vi "[File Management] - PC Module.vi"() -> ()   [LabVIEW 2020]
uses:
  Utility/TypeDefs_Utility/ENUM RB_Pos_Quadrant Position.ctl
  TypeDefs/ENUM_Request PC File Manager.ctl
  TypeDefs/ENUM_State PC File Manager.ctl
  Utility/FP/FPClass/DecFrame_FP/DecFrame_FP.lvclass
  <vilib>/Utility/error.llb/DialogType.ctl
  facef2d7-9603-4ff4-9ff0-56512382c7b7.vi
  d08d4191-17b2-482f-a441-d9d60e68be63.vi
  a00c5825-d05e-4c72-92a9-d0f4f7d392b7.vi
  f268d36e-7cae-4eee-81c7-8a8159c411db.vi
  ade89b95-2dfa-48cf-afe4-b6056d13f73a.vi
  2597e34f-0f19-4283-a693-10768823b2c8.vi
  06699f3f-2e82-4b79-aa69-334e1d5944f8.vi
  <vilib>/Rock Robotics/WPI/ThirdParty/Phoenix-LabVIEW/Motor Controller/Controls/CTRE_Phoenix_MotorControl_TalonFXInvertType.ctl
  Shared Code/TypeDefs/Cluster_Enable-Value DBL.ctl
  <vilib>/Rock Robotics/WPI/ThirdParty/Phoenix-LabVIEW/Motor Controller/Controls/CTRE_Phoenix_MotorControl_NeutralMode.ctl
  Shared Code/TypeDefs/Cluster_Swerve Module Drive Config Data.ctl
  Shared Code/TypeDefs/Cluster_Motion Magic Parameters.ctl
  Shared Code/TypeDefs/Cluster_Swerve Module Azimuth Config Data.ctl
  316f2880-b704-4a84-a7ff-cf39f3abe56d.vi
  f9576979-38bd-4a02-92ac-858de525dc8c.vi
  <vilib>/WebDAVClient/NI_WebDAV.lvlib
  <vilib>/WebDAVClient/Advanced/SessionHandle.ctl
  Shared Code/TypeDefs/Cluster_High-Low.ctl
  Shared Code/TypeDefs/Cluster_PID Gains.ctl
  Shared Code/TypeDefs/Cluster_PID Config.ctl
  Shared Code/TypeDefs/Cluster_Sholder_Config HW Values.ctl
  Shared Code/TypeDefs/Cluster_Extend_Config HW Values.ctl
  Shared Code/TypeDefs/Cluster_Wrist_Config HW Values.ctl
  Shared Code/TypeDefs/ENUM_Motor Index.ctl
  Shared Code/TypeDefs/Cluster_Module Specific Config Data.ctl
  Shared Code/TypeDefs/Cluster_Swerve Specific Data.ctl
  8aa61b50-d4c1-4d7c-b518-7e7f89ee47b3.vi
  293a5106-20bb-4168-be9a-18547983b4f2.vi
  ae0c41dc-fba3-4b78-a09b-fb6d66dd20f7.vi
  fc6d8c50-d7f1-4b91-8983-8391aab75057.vi
  d093f6e5-c98f-44c5-8e41-37ffdc5fbdf3.vi
  Shared Code/TypeDefs/Cluster_Grabber_Config FX Values.ctl
  3a4f407e-2c67-43cb-a4fb-f8418298715f.vi
  <vilib>/WebDAVClient/Advanced/FileInfo.ctl
  d1a17949-e99a-4e11-84fa-4c63115c30d4.vi
  7235e565-7edd-4e1e-80f2-698df6b339dd.vi
  135ee32a-b968-4bc4-aa5f-92b1bd27fa7a.vi
  d92062e0-e931-44ed-a5ae-2fad103b160f.vi
  392f1fec-bdba-4268-92de-5fc60040c1a5.vi
  5390630c-9484-4680-9f8f-9f3095daa9a3.vi
  8e06bce4-31bf-4e2c-9356-0233bb58fc1e.vi
  8021acdc-735e-4c3a-8370-c2cd77d975ff.vi
  fe44edcd-002d-483e-8bc4-2119d9f98af6.vi
  213a5e39-b7ba-45fa-89ff-ac0bf8954cfe.vi
  32e82365-4a9b-4a03-b1c6-655977ec55ce.vi
  6dfe48be-dd7d-41aa-9213-7bde1fbabe93.vi
  ec83e26c-9f45-47fe-bb3a-23606bf88b00.vi
  fc97c97f-c470-4d18-867d-310d18e3dab9.vi
  6ebbc37a-f38e-4f02-af33-7071d1f24c56.vi
  bb6ae5b7-7e89-4e26-bd0e-9cffb8a8ccf7.vi
  Shared Code/TypeDefs/Cluster_FWD  REV Values.ctl
  Shared Code/TypeDefs/Cluster_Config Motor Output.ctl
  Shared Code/TypeDefs/Cluser_Enable-Value I32.ctl
  Shared Code/TypeDefs/Cluser_Config_Soft Limits.ctl
  <vilib>/Rock Robotics/WPI/ThirdParty/Phoenix-LabVIEW/Motor Controller/Controls/CTRE_Phoenix_MotorControl_LimitSwitchNormal.ctl
  Shared Code/TypeDefs/Cluser_Hard Limits.ctl
  Shared Code/TypeDefs/Cluser_Limit Travel Config.ctl
  Shared Code/TypeDefs/Cluser_CAN Data.ctl
  Shared Code/TypeDefs/Cluster_Extend_Config SW Values.ctl
  Shared Code/TypeDefs/Cluser_Config_Current Limits.ctl
  Shared Code/TypeDefs/Cluster_Config_Cancoder Data.ctl
  33df8094-f942-4665-8c4a-d95e8868fd54.vi
  1feea5ea-1d58-47d3-a6aa-f7318612a923.vi
  Shared Code/TypeDefs/ENUM_AutoSelect.ctl
  roboRIO Code/Systems/AUTO 2023/ENUM_CMD_State.ctl
  roboRIO Code/Systems/AUTO 2023/2023-Auto_CMD.lvlib
  roboRIO Code/Systems/AUTO 2023/ENUM_Drive Mode Select.ctl
  Shared Code/TypeDefs/ENUM_Grabber_CMD_Mode Select.ctl
  roboRIO Code/Systems/MotionMaser/ENUM_Pose List.ctl
  roboRIO Code/Systems/MotionMaser/MotionMaster_SubCMD.lvlib
  Shared Code/TypeDefs/Dial_Compase heading unit circle CCW positive.ctl
  Shared Code/TypeDefs/Cluster_Auto Sequence Settings.ctl
  Shared Code/TypeDefs/Cluster_Auto Sequence Data.ctl
  Shared Code/TypeDefs/Cluster_AutoSequence.ctl
  Shared Code/TypeDefs/Cluster_Config_AutoData.ctl
panel:
  in  "AutoData":T1 {"Sequences"."List"."CMDs"."Auto Angle" scale format="%.3f"}
  out "Config NOT Equal":bool
  out "PC Config NOT Saved":bool
  in  "Save RIO Config":bool
  in  "Save PC Config":bool
  in  "Read RIO Config":bool
  in  "Read PC Config":bool
  in  "Copy RIO to PC":bool
  in  "Copy PC to RIO":bool
  in  "Config Tab":T11(tab)
  in  "PC Module Specific Data":T12={"SpecificData Ver"=0, "Data"=[{"Motor Pos"=enum."Left-Front", "CAN Bus"="", "Drive ID"=5, "Azimuth ID"=1, "CanCoder ID"=1, "CanCoder Offset"=14.502}, {"Motor Pos"=enum."Right-Front", "CAN Bus"="", "Drive ID"=6, "Azimuth ID"=2, "CanCoder ID"=2, "CanCoder Offset"=166.816}, {"Motor Pos"=enum."Right-Back", "CAN Bus"="", "Drive ID"=7, "Azimuth ID"=3, "CanCoder ID"=3, "CanCoder Offset"=50.273}, {"Motor Pos"=enum."Left-Back", "CAN Bus"="", "Drive ID"=8, "Azimuth ID"=4, "CanCoder ID"=4, "CanCoder Offset"=332.842}]}
  out "RIO Module Specific Data":T12={"SpecificData Ver"=0, "Data"=[{"Motor Pos"=enum."Left-Front", "CAN Bus"="", "Drive ID"=5, "Azimuth ID"=1, "CanCoder ID"=1, "CanCoder Offset"=14.502}, {"Motor Pos"=enum."Right-Front", "CAN Bus"="", "Drive ID"=6, "Azimuth ID"=2, "CanCoder ID"=2, "CanCoder Offset"=166.816}, {"Motor Pos"=enum."Right-Back", "CAN Bus"="", "Drive ID"=7, "Azimuth ID"=3, "CanCoder ID"=3, "CanCoder Offset"=50.273}, {"Motor Pos"=enum."Left-Back", "CAN Bus"="", "Drive ID"=8, "Azimuth ID"=4, "CanCoder ID"=4, "CanCoder Offset"=332.842}]}
  in  "PC Azimuth Config Data":T15={"ModuleAzimuth Ver"=0, "Output"={"Type"=enum."Clockwise", "Neutral"=enum."Override to Brake", "Max"={"FWD"=0.0, "REV"=2.0}, "Min"={"FWD"=0.0, "REV"=0.0}, "OL Ramp Rate (S)"=0.0, "Dead Band"=0.0}, "CL"={"Gains"={"P"=0.0, "I"=0.0, "D"=20.0, "F"=0.0}, "Error Allowed"={"High"=0.0, "Low"=0.0}, "I Zone"={"High"=0.0, "Low"=0.0}, "Max Out"={"FWD"=20.0, "REV"=0.0}, "Max I Accu"={"High"=1.0, "Low"=-1.0}, "CL Ramp Rate (S)"=0.0}, "MM"={"Cruise Velocity"=0, "Acceleration"=0}} {"Output"."Min"."REV" format="%.2f"; "Output"."Min"."FWD" format="%.2f"; "Output"."Max"."REV" format="%.2f"; "Output"."Max"."FWD" format="%.2f"; "CL"."Max I Accu"."Low" format="%#.8f"; "CL"."Max I Accu"."High" format="%#.8f"; "CL"."Gains"."F" format="%#.8f"; "CL"."Gains"."D" format="%#.8f"; "CL"."Gains"."I" format="%#.8f"; "CL"."Gains"."P" format="%#.8f"; "CL"."Error Allowed"."Low" format="%#.8f"; "CL"."Error Allowed"."High" format="%#.8f"; "CL"."I Zone"."Low" format="%#.8f"; "CL"."I Zone"."High" format="%#.8f"; "CL"."Max Out"."REV" format="%.2f"; "CL"."Max Out"."FWD" format="%.2f"}
  out "RIO Azimuth Config Data":T15={"ModuleAzimuth Ver"=0, "Output"={"Type"=enum."Clockwise", "Neutral"=enum."Override to Brake", "Max"={"FWD"=0.0, "REV"=2.0}, "Min"={"FWD"=0.0, "REV"=0.0}, "OL Ramp Rate (S)"=0.0, "Dead Band"=0.0}, "CL"={"Gains"={"P"=0.0, "I"=0.0, "D"=20.0, "F"=0.0}, "Error Allowed"={"High"=0.0, "Low"=0.0}, "I Zone"={"High"=0.0, "Low"=0.0}, "Max Out"={"FWD"=20.0, "REV"=0.0}, "Max I Accu"={"High"=1.0, "Low"=-1.0}, "CL Ramp Rate (S)"=0.0}, "MM"={"Cruise Velocity"=0, "Acceleration"=0}} {"Output"."Min"."REV" format="%.2f"; "Output"."Min"."FWD" format="%.2f"; "Output"."Max"."REV" format="%.2f"; "Output"."Max"."FWD" format="%.2f"; "CL"."Max I Accu"."Low" format="%#.8f"; "CL"."Max I Accu"."High" format="%#.8f"; "CL"."Gains"."F" format="%#.8f"; "CL"."Gains"."D" format="%#.8f"; "CL"."Gains"."I" format="%#.8f"; "CL"."Gains"."P" format="%#.8f"; "CL"."Error Allowed"."Low" format="%#.8f"; "CL"."Error Allowed"."High" format="%#.8f"; "CL"."I Zone"."Low" format="%#.8f"; "CL"."I Zone"."High" format="%#.8f"; "CL"."Max Out"."REV" format="%.2f"; "CL"."Max Out"."FWD" format="%.2f"}
  in  "PC Drive Config Data":T24={"ModuleDrive Ver"=0, "Output"={"Type"=enum."Counter-Clockwise", "Neutral"=enum."EEPROMSetting", "Max"={"FWD"=0.0, "REV"=0.0}, "Min"={"FWD"=0.0, "REV"=0.0}, "OL Ramp Rate (S)"=0.0, "Dead Band"=0.0}, "CL"={"Gains"={"P"=1.0, "I"=0.01, "D"=0.0, "F"=0.0}, "Error Allowed"={"High"=0.1, "Low"=-0.1}, "I Zone"={"High"=10.0, "Low"=-10.0}, "Max Out"={"FWD"=100.0, "REV"=-100.0}, "Max I Accu"={"High"=0.0, "Low"=0.0}, "CL Ramp Rate (S)"=0.0}, "VoltageComp"={"Enable"=FALSE, "Value"=0.0}} {"Output"."Min"."REV" format="%.2f"; "Output"."Min"."FWD" format="%.2f"; "Output"."Max"."REV" format="%.2f"; "Output"."Max"."FWD" format="%.2f"; "VoltageComp"."Value" format="%.1g"; "CL"."Max I Accu"."Low" format="%#.8f"; "CL"."Max I Accu"."High" format="%#.8f"; "CL"."Gains"."F" format="%#.8f"; "CL"."Gains"."D" format="%#.8f"; "CL"."Gains"."I" format="%#.8f"; "CL"."Gains"."P" format="%#.8f"; "CL"."Error Allowed"."Low" format="%#.8f"; "CL"."Error Allowed"."High" format="%#.8f"; "CL"."I Zone"."Low" format="%#.8f"; "CL"."I Zone"."High" format="%#.8f"; "CL"."Max Out"."REV" format="%.2f"; "CL"."Max Out"."FWD" format="%.2f"}
  out "RIO Drive Config Data":T24={"ModuleDrive Ver"=0, "Output"={"Type"=enum."Counter-Clockwise", "Neutral"=enum."EEPROMSetting", "Max"={"FWD"=0.0, "REV"=0.0}, "Min"={"FWD"=0.0, "REV"=0.0}, "OL Ramp Rate (S)"=0.0, "Dead Band"=0.0}, "CL"={"Gains"={"P"=1.0, "I"=0.01, "D"=0.0, "F"=0.0}, "Error Allowed"={"High"=0.1, "Low"=-0.1}, "I Zone"={"High"=10.0, "Low"=-10.0}, "Max Out"={"FWD"=100.0, "REV"=-100.0}, "Max I Accu"={"High"=0.0, "Low"=0.0}, "CL Ramp Rate (S)"=0.0}, "VoltageComp"={"Enable"=FALSE, "Value"=0.0}} {"Output"."Min"."REV" format="%.2f"; "Output"."Min"."FWD" format="%.2f"; "Output"."Max"."REV" format="%.2f"; "Output"."Max"."FWD" format="%.2f"; "VoltageComp"."Value" format="%.1g"; "CL"."Max I Accu"."Low" format="%#.8f"; "CL"."Max I Accu"."High" format="%#.8f"; "CL"."Gains"."F" format="%#.8f"; "CL"."Gains"."D" format="%#.8f"; "CL"."Gains"."I" format="%#.8f"; "CL"."Gains"."P" format="%#.8f"; "CL"."Error Allowed"."Low" format="%#.8f"; "CL"."Error Allowed"."High" format="%#.8f"; "CL"."I Zone"."Low" format="%#.8f"; "CL"."I Zone"."High" format="%#.8f"; "CL"."Max Out"."REV" format="%.2f"; "CL"."Max Out"."FWD" format="%.2f"}
  in  "PC Sholder Config":T26={"SholderHW Ver"=0, "CAN"={"ID"=0, "Bus"=""}, "Output"={"Type"=enum."Counter-Clockwise", "Neutral"=enum."Override to Brake", "Max"={"FWD"=0.0, "REV"=-1.0}, "Min"={"FWD"=0.0, "REV"=0.0}, "OL Ramp Rate (S)"=0.0, "Dead Band"=0.0}, "CL"={"Gains"={"P"=1.0, "I"=0.01, "D"=0.0, "F"=0.0}, "Error Allowed"={"High"=0.0, "Low"=0.0}, "I Zone"={"High"=10000.0, "Low"=-1000.0}, "Max Out"={"FWD"=1.0, "REV"=-1.0}, "Max I Accu"={"High"=10.0, "Low"=-10.0}, "CL Ramp Rate (S)"=0.0}, "MM"={"Cruise Velocity"=5000, "Acceleration"=5000}, "TravelLimits"={"Hard"={"FWD Switch Normal"=enum."Normally Open", "FWD On will Zero Encoder "=FALSE, "REV Switch Normal"=enum."Normally Open", "REV On will Zero Encoder "=FALSE}, "Soft"={"FWD"={"Enable"=FALSE, "Counts"=0}, "REV"={"Enable"=FALSE, "Counts"=0}}}, "Cancoder"={"ID"=0, "CW(t) CCW(f)"=TRUE, "Zero Offset"=0.0}} {"TravelLimits"."Soft"."REV"."Counts" format="%#.0f"; "TravelLimits"."Soft"."FWD"."Counts" format="%#.0f"; "Output"."Min"."REV" format="%.2f"; "Output"."Min"."FWD" format="%.2f"; "Output"."Max"."REV" format="%.2f"; "Output"."Max"."FWD" format="%.2f"; "CL"."Max I Accu"."Low" format="%#.8f"; "CL"."Max I Accu"."High" format="%#.8f"; "CL"."Gains"."F" format="%#.8f"; "CL"."Gains"."D" format="%#.8f"; "CL"."Gains"."I" format="%#.8f"; "CL"."Gains"."P" format="%#.8f"; "CL"."Error Allowed"."Low" format="%#.8f"; "CL"."Error Allowed"."High" format="%#.8f"; "CL"."I Zone"."Low" format="%#.8f"; "CL"."I Zone"."High" format="%#.8f"; "CL"."Max Out"."REV" format="%.2f"; "CL"."Max Out"."FWD" format="%.2f"}
  out "RIO Sholder Config":T26={"SholderHW Ver"=0, "CAN"={"ID"=0, "Bus"=""}, "Output"={"Type"=enum."Counter-Clockwise", "Neutral"=enum."Override to Brake", "Max"={"FWD"=0.0, "REV"=-1.0}, "Min"={"FWD"=0.0, "REV"=0.0}, "OL Ramp Rate (S)"=0.0, "Dead Band"=0.0}, "CL"={"Gains"={"P"=1.0, "I"=0.01, "D"=0.0, "F"=0.0}, "Error Allowed"={"High"=0.0, "Low"=0.0}, "I Zone"={"High"=10000.0, "Low"=-1000.0}, "Max Out"={"FWD"=1.0, "REV"=-1.0}, "Max I Accu"={"High"=10.0, "Low"=-10.0}, "CL Ramp Rate (S)"=0.0}, "MM"={"Cruise Velocity"=5000, "Acceleration"=5000}, "TravelLimits"={"Hard"={"FWD Switch Normal"=enum."Normally Open", "FWD On will Zero Encoder "=FALSE, "REV Switch Normal"=enum."Normally Open", "REV On will Zero Encoder "=FALSE}, "Soft"={"FWD"={"Enable"=FALSE, "Counts"=0}, "REV"={"Enable"=FALSE, "Counts"=0}}}, "Cancoder"={"ID"=0, "CW(t) CCW(f)"=TRUE, "Zero Offset"=0.0}} {"TravelLimits"."Soft"."REV"."Counts" format="%#.0f"; "TravelLimits"."Soft"."FWD"."Counts" format="%#.0f"; "Output"."Min"."REV" format="%.2f"; "Output"."Min"."FWD" format="%.2f"; "Output"."Max"."REV" format="%.2f"; "Output"."Max"."FWD" format="%.2f"; "CL"."Max I Accu"."Low" format="%#.8f"; "CL"."Max I Accu"."High" format="%#.8f"; "CL"."Gains"."F" format="%#.8f"; "CL"."Gains"."D" format="%#.8f"; "CL"."Gains"."I" format="%#.8f"; "CL"."Gains"."P" format="%#.8f"; "CL"."Error Allowed"."Low" format="%#.8f"; "CL"."Error Allowed"."High" format="%#.8f"; "CL"."I Zone"."Low" format="%#.8f"; "CL"."I Zone"."High" format="%#.8f"; "CL"."Max Out"."REV" format="%.2f"; "CL"."Max Out"."FWD" format="%.2f"}
  in  "PC Extend ConfigFX":T34={"ExtendHW Ver"=0, "CAN"={"ID"=0, "Bus"=""}, "Output"={"Type"=enum."Counter-Clockwise", "Neutral"=enum."Override to Brake", "Max"={"FWD"=0.0, "REV"=-1.0}, "Min"={"FWD"=0.0, "REV"=0.0}, "OL Ramp Rate (S)"=0.0, "Dead Band"=0.0}, "CL"={"Gains"={"P"=1.0, "I"=0.01, "D"=0.0, "F"=0.0}, "Error Allowed"={"High"=0.0, "Low"=0.0}, "I Zone"={"High"=10000.0, "Low"=-1000.0}, "Max Out"={"FWD"=1.0, "REV"=-1.0}, "Max I Accu"={"High"=10.0, "Low"=-10.0}, "CL Ramp Rate (S)"=0.0}, "MM"={"Cruise Velocity"=5000, "Acceleration"=5000}, "TravelLimits"={"Hard"={"FWD Switch Normal"=enum."Normally Open", "FWD On will Zero Encoder "=FALSE, "REV Switch Normal"=enum."Normally Open", "REV On will Zero Encoder "=FALSE}, "Soft"={"FWD"={"Enable"=FALSE, "Counts"=0}, "REV"={"Enable"=FALSE, "Counts"=0}}}, "StatorLimit"={"Enable"=FALSE, "Current Limit"=0.0, "Threshold Current"=0.0, "Threshold Time"=0.0}, "Cancoder"={"ID"=0, "CW(t) CCW(f)"=FALSE, "Zero Offset"=0.0}} {"TravelLimits"."Soft"."REV"."Counts" format="%#.0f"; "TravelLimits"."Soft"."FWD"."Counts" format="%#.0f"; "Output"."Min"."REV" format="%.2f"; "Output"."Min"."FWD" format="%.2f"; "Output"."Max"."REV" format="%.2f"; "Output"."Max"."FWD" format="%.2f"; "CL"."Max I Accu"."Low" format="%#.8f"; "CL"."Max I Accu"."High" format="%#.8f"; "CL"."Gains"."F" format="%#.8f"; "CL"."Gains"."D" format="%#.8f"; "CL"."Gains"."I" format="%#.8f"; "CL"."Gains"."P" format="%#.8f"; "CL"."Error Allowed"."Low" format="%#.8f"; "CL"."Error Allowed"."High" format="%#.8f"; "CL"."I Zone"."Low" format="%#.8f"; "CL"."I Zone"."High" format="%#.8f"; "CL"."Max Out"."REV" format="%.2f"; "CL"."Max Out"."FWD" format="%.2f"}
  out "RIO Extender Config":T34={"ExtendHW Ver"=0, "CAN"={"ID"=0, "Bus"=""}, "Output"={"Type"=enum."Counter-Clockwise", "Neutral"=enum."Override to Brake", "Max"={"FWD"=0.0, "REV"=-1.0}, "Min"={"FWD"=0.0, "REV"=0.0}, "OL Ramp Rate (S)"=0.0, "Dead Band"=0.0}, "CL"={"Gains"={"P"=1.0, "I"=0.01, "D"=0.0, "F"=0.0}, "Error Allowed"={"High"=0.0, "Low"=0.0}, "I Zone"={"High"=10000.0, "Low"=-1000.0}, "Max Out"={"FWD"=1.0, "REV"=-1.0}, "Max I Accu"={"High"=10.0, "Low"=-10.0}, "CL Ramp Rate (S)"=0.0}, "MM"={"Cruise Velocity"=5000, "Acceleration"=5000}, "TravelLimits"={"Hard"={"FWD Switch Normal"=enum."Normally Open", "FWD On will Zero Encoder "=FALSE, "REV Switch Normal"=enum."Normally Open", "REV On will Zero Encoder "=FALSE}, "Soft"={"FWD"={"Enable"=FALSE, "Counts"=0}, "REV"={"Enable"=FALSE, "Counts"=0}}}, "StatorLimit"={"Enable"=FALSE, "Current Limit"=0.0, "Threshold Current"=0.0, "Threshold Time"=0.0}, "Cancoder"={"ID"=0, "CW(t) CCW(f)"=FALSE, "Zero Offset"=0.0}} {"TravelLimits"."Soft"."REV"."Counts" format="%#.0f"; "TravelLimits"."Soft"."FWD"."Counts" format="%#.0f"; "Output"."Min"."REV" format="%.2f"; "Output"."Min"."FWD" format="%.2f"; "Output"."Max"."REV" format="%.2f"; "Output"."Max"."FWD" format="%.2f"; "CL"."Max I Accu"."Low" format="%#.8f"; "CL"."Max I Accu"."High" format="%#.8f"; "CL"."Gains"."F" format="%#.8f"; "CL"."Gains"."D" format="%#.8f"; "CL"."Gains"."I" format="%#.8f"; "CL"."Gains"."P" format="%#.8f"; "CL"."Error Allowed"."Low" format="%#.8f"; "CL"."Error Allowed"."High" format="%#.8f"; "CL"."I Zone"."Low" format="%#.8f"; "CL"."I Zone"."High" format="%#.8f"; "CL"."Max Out"."REV" format="%.2f"; "CL"."Max Out"."FWD" format="%.2f"}
  in  "PC Wrist Config":T36={"WristHW Ver"=0, "CAN"={"ID"=0, "Bus"=""}, "Output"={"Type"=enum."Counter-Clockwise", "Neutral"=enum."Override to Brake", "Max"={"FWD"=0.0, "REV"=-1.0}, "Min"={"FWD"=0.0, "REV"=0.0}, "OL Ramp Rate (S)"=0.0, "Dead Band"=0.0}, "CL"={"Gains"={"P"=1.0, "I"=0.01, "D"=0.0, "F"=0.0}, "Error Allowed"={"High"=0.0, "Low"=0.0}, "I Zone"={"High"=10000.0, "Low"=-1000.0}, "Max Out"={"FWD"=1.0, "REV"=-1.0}, "Max I Accu"={"High"=10.0, "Low"=-10.0}, "CL Ramp Rate (S)"=0.0}, "MM"={"Cruise Velocity"=5000, "Acceleration"=5000}, "TravelLimits"={"Hard"={"FWD Switch Normal"=enum."Normally Open", "FWD On will Zero Encoder "=FALSE, "REV Switch Normal"=enum."Normally Open", "REV On will Zero Encoder "=FALSE}, "Soft"={"FWD"={"Enable"=FALSE, "Counts"=0}, "REV"={"Enable"=FALSE, "Counts"=0}}}, "Cancoder"={"ID"=0, "CW(t) CCW(f)"=TRUE, "Zero Offset"=0.0}, "CurrentLimit"={"Enable"=FALSE, "Current Limit"=0.0, "Threshold Current"=0.0, "Threshold Time"=0.0}} {"TravelLimits"."Soft"."REV"."Counts" format="%#.0f"; "TravelLimits"."Soft"."FWD"."Counts" format="%#.0f"; "Output"."Min"."REV" format="%.2f"; "Output"."Min"."FWD" format="%.2f"; "Output"."Max"."REV" format="%.2f"; "Output"."Max"."FWD" format="%.2f"; "CL"."Max I Accu"."Low" format="%#.8f"; "CL"."Max I Accu"."High" format="%#.8f"; "CL"."Gains"."F" format="%#.8f"; "CL"."Gains"."D" format="%#.8f"; "CL"."Gains"."I" format="%#.8f"; "CL"."Gains"."P" format="%#.8f"; "CL"."Error Allowed"."Low" format="%#.8f"; "CL"."Error Allowed"."High" format="%#.8f"; "CL"."I Zone"."Low" format="%#.8f"; "CL"."I Zone"."High" format="%#.8f"; "CL"."Max Out"."REV" format="%.2f"; "CL"."Max Out"."FWD" format="%.2f"}
  out "RIO Wrist Config":T36={"WristHW Ver"=0, "CAN"={"ID"=0, "Bus"=""}, "Output"={"Type"=enum."Counter-Clockwise", "Neutral"=enum."Override to Brake", "Max"={"FWD"=0.0, "REV"=-1.0}, "Min"={"FWD"=0.0, "REV"=0.0}, "OL Ramp Rate (S)"=0.0, "Dead Band"=0.0}, "CL"={"Gains"={"P"=1.0, "I"=0.01, "D"=0.0, "F"=0.0}, "Error Allowed"={"High"=0.0, "Low"=0.0}, "I Zone"={"High"=10000.0, "Low"=-1000.0}, "Max Out"={"FWD"=1.0, "REV"=-1.0}, "Max I Accu"={"High"=10.0, "Low"=-10.0}, "CL Ramp Rate (S)"=0.0}, "MM"={"Cruise Velocity"=5000, "Acceleration"=5000}, "TravelLimits"={"Hard"={"FWD Switch Normal"=enum."Normally Open", "FWD On will Zero Encoder "=FALSE, "REV Switch Normal"=enum."Normally Open", "REV On will Zero Encoder "=FALSE}, "Soft"={"FWD"={"Enable"=FALSE, "Counts"=0}, "REV"={"Enable"=FALSE, "Counts"=0}}}, "Cancoder"={"ID"=0, "CW(t) CCW(f)"=TRUE, "Zero Offset"=0.0}, "CurrentLimit"={"Enable"=FALSE, "Current Limit"=0.0, "Threshold Current"=0.0, "Threshold Time"=0.0}} {"TravelLimits"."Soft"."REV"."Counts" format="%#.0f"; "TravelLimits"."Soft"."FWD"."Counts" format="%#.0f"; "Output"."Min"."REV" format="%.2f"; "Output"."Min"."FWD" format="%.2f"; "Output"."Max"."REV" format="%.2f"; "Output"."Max"."FWD" format="%.2f"; "CL"."Max I Accu"."Low" format="%#.8f"; "CL"."Max I Accu"."High" format="%#.8f"; "CL"."Gains"."F" format="%#.8f"; "CL"."Gains"."D" format="%#.8f"; "CL"."Gains"."I" format="%#.8f"; "CL"."Gains"."P" format="%#.8f"; "CL"."Error Allowed"."Low" format="%#.8f"; "CL"."Error Allowed"."High" format="%#.8f"; "CL"."I Zone"."Low" format="%#.8f"; "CL"."I Zone"."High" format="%#.8f"; "CL"."Max Out"."REV" format="%.2f"; "CL"."Max Out"."FWD" format="%.2f"}
  in  "PC ExtendProgram Config":T37={"ExtendSW Ver"=0, "Home Speed (0-1)"=0.0, "Enable Current Limit On Homing"=FALSE, "At Position Delay(S)"=0.2}
  out "RIO ExtendProgram Config":T37={"ExtendSW Ver"=0, "Home Speed (0-1)"=0.0, "Enable Current Limit On Homing"=FALSE, "At Position Delay(S)"=0.2}
  in  "PC Grabber Config":T38={"Grabber Ver"=0, "CAN"={"ID"=136, "Bus"=""}, "Output"={"Type"=enum."Counter-Clockwise", "Neutral"=enum."Override to Brake", "Max"={"FWD"=0.0, "REV"=5000.0}, "Min"={"FWD"=0.0, "REV"=0.0}, "OL Ramp Rate (S)"=0.0, "Dead Band"=0.0}, "StatorLimit"={"Enable"=FALSE, "Current Limit"=0.0, "Threshold Current"=0.0, "Threshold Time"=0.0}} {"Output"."Min"."REV" format="%.2f"; "Output"."Min"."FWD" format="%.2f"; "Output"."Max"."REV" format="%.2f"; "Output"."Max"."FWD" format="%.2f"}
  out "RIO Grabber Config":T38={"Grabber Ver"=0, "CAN"={"ID"=136, "Bus"=""}, "Output"={"Type"=enum."Counter-Clockwise", "Neutral"=enum."Override to Brake", "Max"={"FWD"=0.0, "REV"=5000.0}, "Min"={"FWD"=0.0, "REV"=0.0}, "OL Ramp Rate (S)"=0.0, "Dead Band"=0.0}, "StatorLimit"={"Enable"=FALSE, "Current Limit"=0.0, "Threshold Current"=0.0, "Threshold Time"=0.0}} {"Output"."Min"."REV" format="%.2f"; "Output"."Min"."FWD" format="%.2f"; "Output"."Max"."REV" format="%.2f"; "Output"."Max"."FWD" format="%.2f"}
  out "PC Folder Found":bool
  out "RIO Folder Found":bool
  out "RIO Connected":bool
  out "PC Folder Path":path
  in  "RIO Folder Path":string
  in  "Select":bool[](array[boolean])
  in  "RIO IP List":string[](array[string])
  out "Message":string
  in  "stop":bool
  out "Action":string
  out "Next Request":T39 caption="Request"
  out "State":T40=enum."Connecting to RIO"
  # "Tune Output\nto 1023 Max"
  # "Tune Output\nto 1023 Max"
  # "Tune to Output\nto 1023 Max"
  # "Tune to Output\nto 1023 Max"
  # "Tune Output\nto 1023 Max"
  # "Tune Output\nto 1023 Max"
  # "Tune Output\nto 1023 Max"
  # "Tune Output\nto 1023 Max"
  # "Tune Output\nto 1023 Max"
  # "Tune Output\nto 1023 Max"
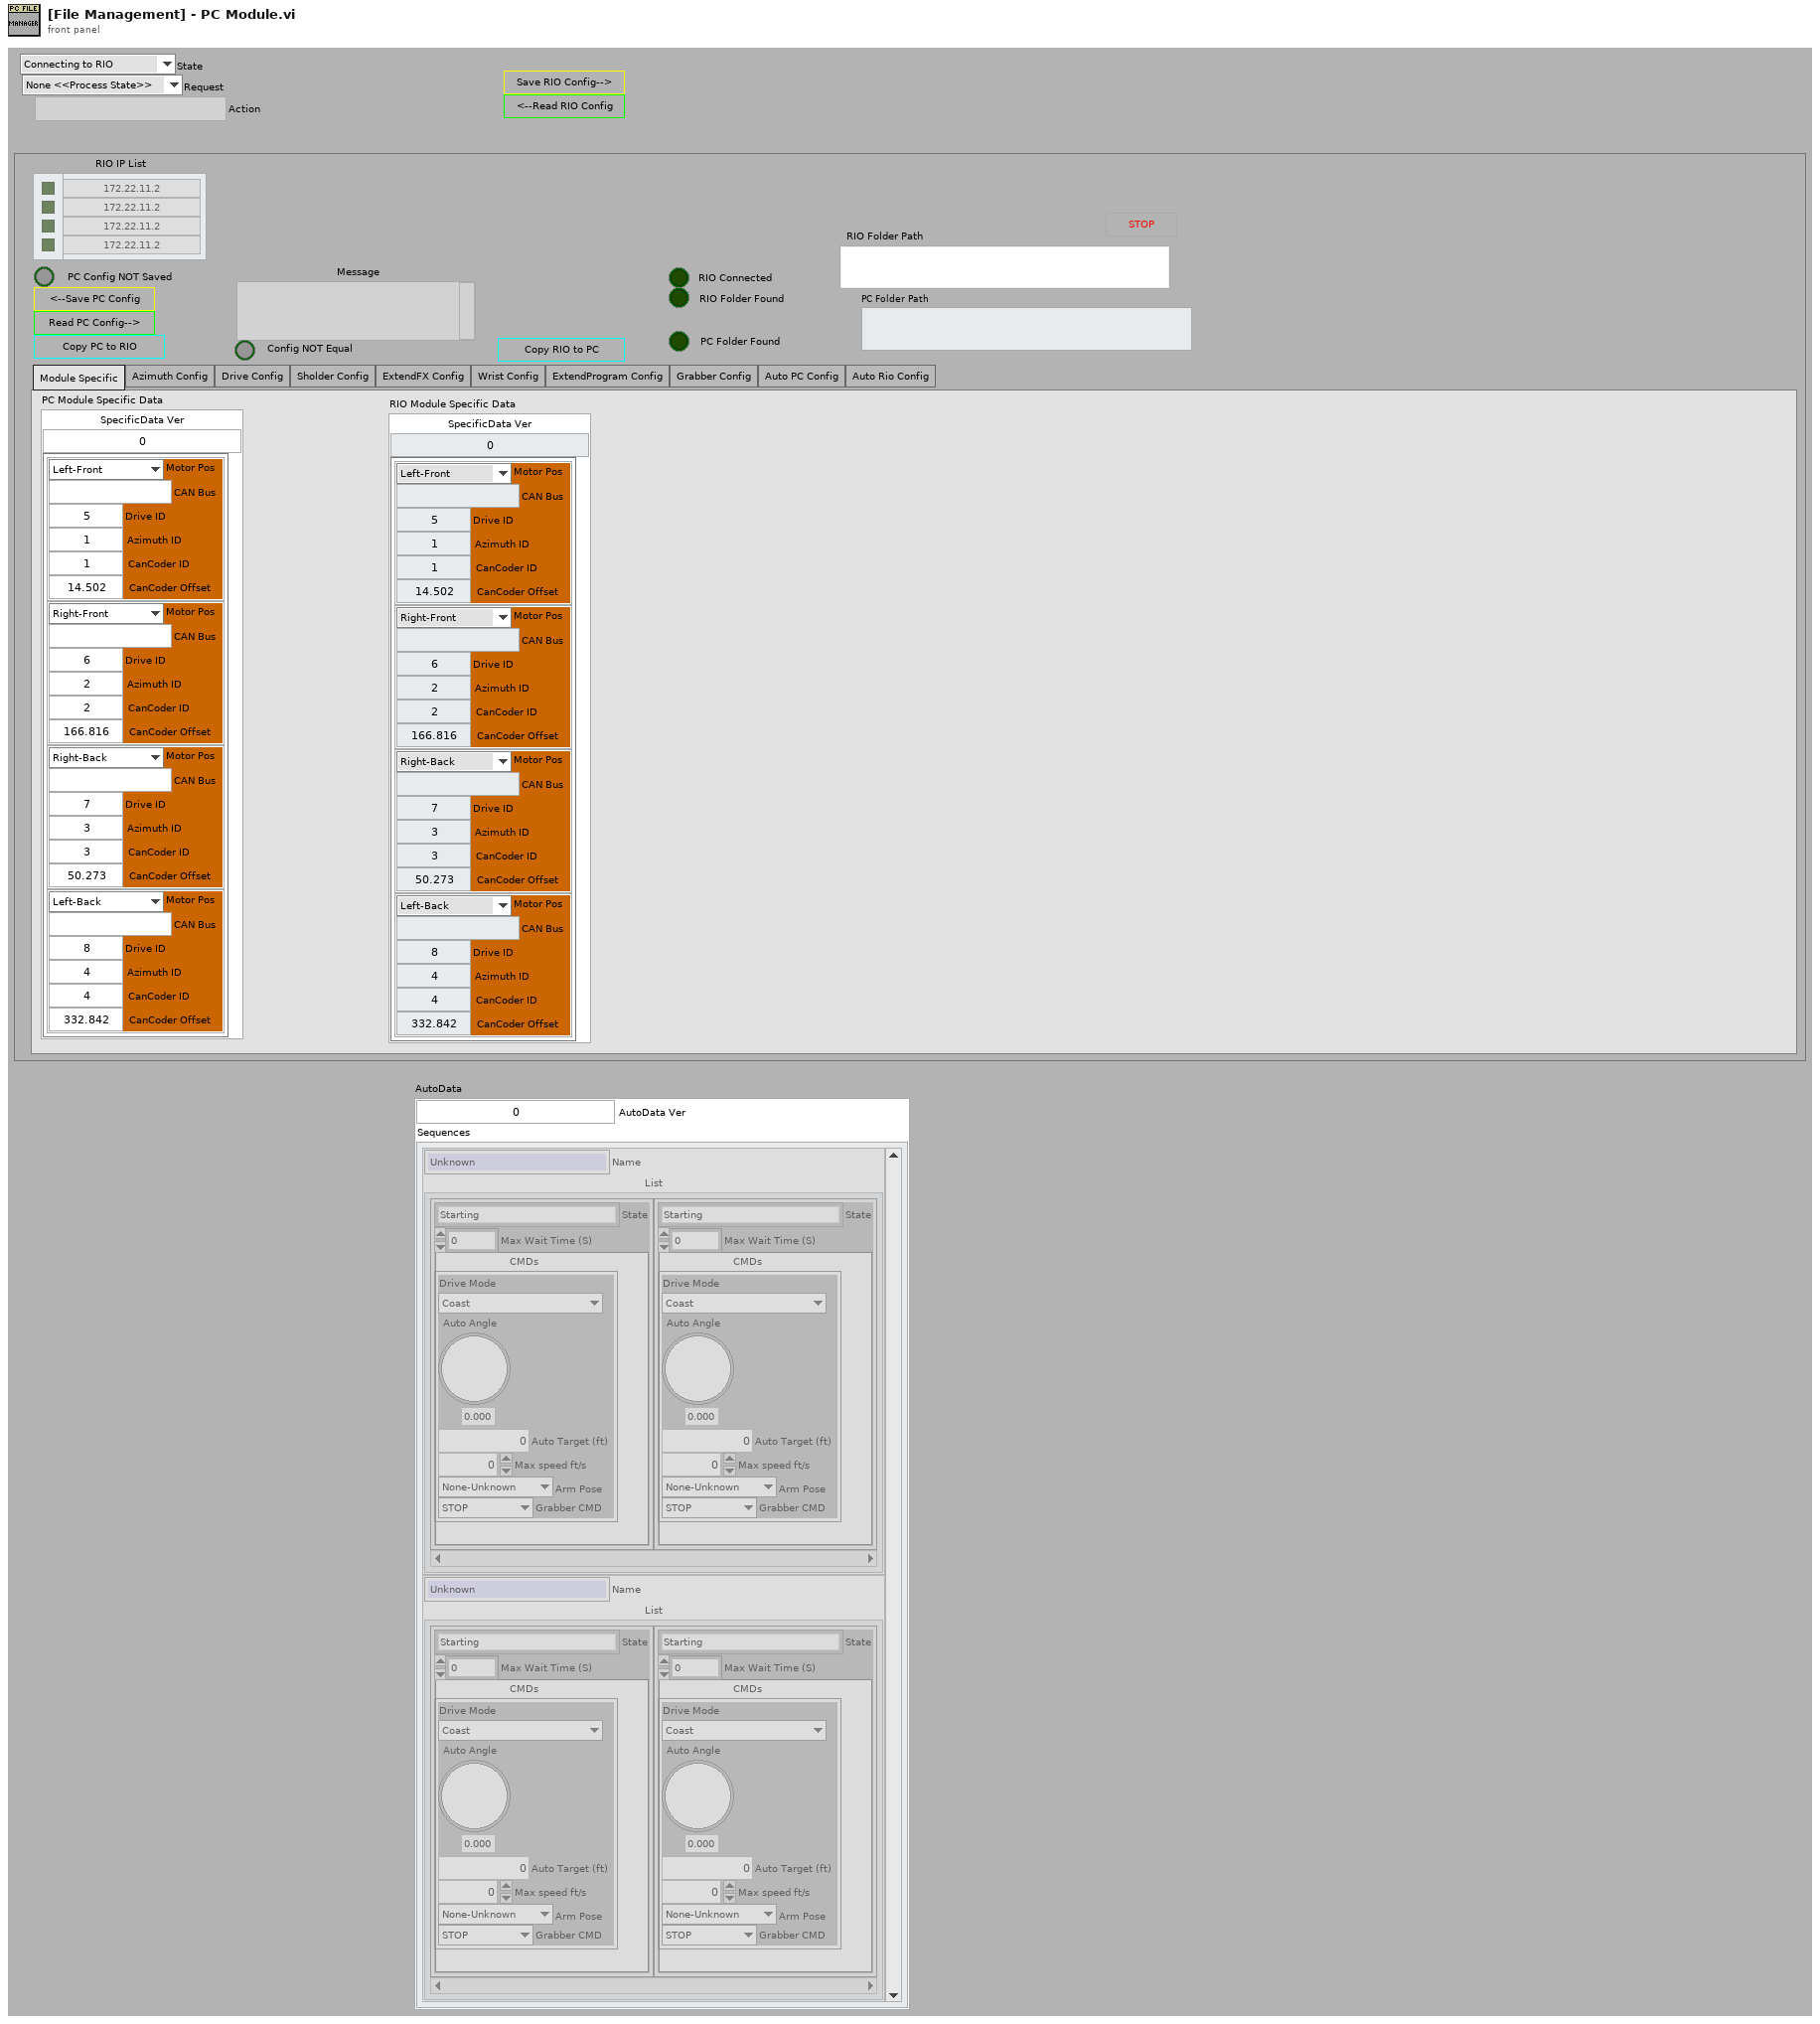
[diagram p1: front panel]
types:
  T1 = typedef "Cluster_Config_AutoData.ctl" = cluster{"AutoData Ver":u64, "Sequences":T2[]}
  T2 = typedef "Cluster_AutoSequence.ctl" = cluster{"Name":T3, "List":T4[]}
  T3 = typedef "ENUM_AutoSelect.ctl" = enum16{"Unknown", "Drop Mid Drive Straight", "Drop mid dock and engage", "Drop High dock and engage", "Drop Low dock and engage", "Manual", "Over and Rebalance", "Over and Dock", "Score Mid Over and Balance", "Score High Over and Balance", "Score Mid ONLY", "Score High ONLY"}
  T4 = typedef "Cluster_Auto Sequence Data.ctl" = cluster{"State":T5, "Max Wait Time (S)":dbl, "CMDs":T6, "Color Box":u32}
  T5 = typedef "2023-Auto_CMD.lvlib/ENUM_CMD_State.ctl" = enum16{"Starting", "Idling", "Selecting Sequence", "Selecting Next Step", "Driving to Position", "Stopping", "Grabbing", "Moving Arm", "Rotation Target", "Waiting", "Shutting Down", "Balancing Level", "Configuring", "Tilt UP or Position", "Tile DOWN or Position", "LEVEL or Position"}
  T6 = typedef "Cluster_Auto Sequence Settings.ctl" = cluster{"Drive Mode":T7, "Auto Angle":T8, "Auto Target (ft)":dbl, "Max speed ft/s":dbl, "Arm Pose ":T9, "Grabber CMD":T10}
  T7 = typedef "2023-Auto_CMD.lvlib/ENUM_Drive Mode Select.ctl" = enum16{"Coast", "To Position", "Rotation Absolute", "Balance on Charger", "Brake", "Lock"}
  T8 = typedef "Dial_Compase heading unit circle CCW positive.ctl" = dbl
  T9 = typedef "MotionMaster_SubCMD.lvlib/ENUM_Pose List.ctl" = enum16{"None-Unknown", "Intake", "Score High", "Score Mid", "Safe Position", "Home Pos"}
  T10 = typedef "ENUM_Grabber_CMD_Mode Select.ctl" = enum16{"STOP", "Intake", "Eject"}
  T11 = enum32{"Module Specific", "Azimuth Config", "Drive Config", "Sholder Config", "ExtendFX Config", "Wrist Config", "ExtendProgram Config", "Grabber Config", "Auto PC Config", "Auto Rio Config"}
  T12 = typedef "Cluster_Swerve Specific Data.ctl" = cluster{"SpecificData Ver":u64, "Data":T13[]}
  T13 = typedef "Cluster_Module Specific Config Data.ctl" = cluster{"Motor Pos":T14, "CAN Bus":string, "Drive ID":u8, "Azimuth ID":u8, "CanCoder ID":u8, "CanCoder Offset":dbl}
  T14 = typedef "ENUM_Motor Index.ctl" = enum16{"Left-Front", "Right-Front", "Left-Back", "Right-Back"}
  T15 = typedef "Cluster_Swerve Module Azimuth Config Data.ctl" = cluster{"ModuleAzimuth Ver":u64, "Output":T16, "CL":T20, "MM":T23}
  T16 = typedef "Cluster_Config Motor Output.ctl" = cluster{"Type":T17, "Neutral":T18, "Max":T19, "Min":T19, "OL Ramp Rate (S)":dbl, "Dead Band":dbl}
  T17 = typedef "CTRE_Phoenix_MotorControl_TalonFXInvertType.ctl" = enum16{"Counter-Clockwise", "Clockwise"}
  T18 = typedef "CTRE_Phoenix_MotorControl_NeutralMode.ctl" = enum8{"EEPROMSetting", "Override to Coast", "Override to Brake"}
  T19 = typedef "Cluster_FWD  REV Values.ctl" = cluster{"FWD":dbl, "REV":dbl}
  T20 = typedef "Cluster_PID Config.ctl" = cluster{"Gains":T21, "Error Allowed":T22, "I Zone":T22, "Max Out":T19, "Max I Accu":T22, "CL Ramp Rate (S)":dbl}
  T21 = typedef "Cluster_PID Gains.ctl" = cluster{"P":dbl, "I":dbl, "D":dbl, "F":dbl}
  T22 = typedef "Cluster_High-Low.ctl" = cluster{"High":dbl, "Low":dbl}
  T23 = typedef "Cluster_Motion Magic Parameters.ctl" = cluster{"Cruise Velocity":i32, "Acceleration":i32}
  T24 = typedef "Cluster_Swerve Module Drive Config Data.ctl" = cluster{"ModuleDrive Ver":u64, "Output":T16, "CL":T20, "VoltageComp":T25}
  T25 = typedef "Cluster_Enable-Value DBL.ctl" = cluster{"Enable":bool, "Value":dbl}
  T26 = typedef "Cluster_Sholder_Config HW Values.ctl" = cluster{"SholderHW Ver":u64, "CAN":T27, "Output":T16, "CL":T20, "MM":T23, "TravelLimits":T28, "Cancoder":T33}
  T27 = typedef "Cluser_CAN Data.ctl" = cluster{"ID":u8, "Bus":string}
  T28 = typedef "Cluser_Limit Travel Config.ctl" = cluster{"Hard":T29, "Soft":T31}
  T29 = typedef "Cluser_Hard Limits.ctl" = cluster{"FWD Switch Normal":T30, "FWD On will Zero Encoder ":bool, "REV Switch Normal":T30, "REV On will Zero Encoder ":bool}
  T30 = typedef "CTRE_Phoenix_MotorControl_LimitSwitchNormal.ctl" = enum16{"Normally Open", "Normally Closed", "Disabled"}
  T31 = typedef "Cluser_Config_Soft Limits.ctl" = cluster{"FWD":T32, "REV":T32}
  T32 = typedef "Cluser_Enable-Value I32.ctl" = cluster{"Enable":bool, "Counts":i32}
  T33 = typedef "Cluster_Config_Cancoder Data.ctl" = cluster{"ID":u8, "CW(t) CCW(f)":bool, "Zero Offset":dbl}
  T34 = typedef "Cluster_Extend_Config HW Values.ctl" = cluster{"ExtendHW Ver":u64, "CAN":T27, "Output":T16, "CL":T20, "MM":T23, "TravelLimits":T28, "StatorLimit":T35, "Cancoder":T33}
  T35 = typedef "Cluser_Config_Current Limits.ctl" = cluster{"Enable":bool, "Current Limit":dbl, "Threshold Current":dbl, "Threshold Time":dbl}
  T36 = typedef "Cluster_Wrist_Config HW Values.ctl" = cluster{"WristHW Ver":u64, "CAN":T27, "Output":T16, "CL":T20, "MM":T23, "TravelLimits":T28, "Cancoder":T33, "CurrentLimit":T35}
  T37 = typedef "Cluster_Extend_Config SW Values.ctl" = cluster{"ExtendSW Ver":u64, "Home Speed (0-1)":dbl, "Enable Current Limit On Homing":bool, "At Position Delay(S)":dbl}
  T38 = typedef "Cluster_Grabber_Config FX Values.ctl" = cluster{"Grabber Ver":u64, "CAN":T27, "Output":T16, "StatorLimit":T35}
  T39 = typedef "ENUM_Request PC File Manager.ctl" = enum16{"None <<Process State>>", "Conect to RIO", "SetFP Request", "Stop Program", "Save PC Config", "Save RIO Config", "Read PC Config", "Read RIO Config", "Tab Change"}
  T40 = typedef "ENUM_State PC File Manager.ctl" = enum16{"<Startup>", "Connecting to RIO", "Waiting for Valid Folder", "Waiting for Instruction", "<Shutdown>"}
  T41 = typedef "NI_WebDAV.lvlib/FileInfo.ctl" = cluster{"type":string, "size":u64, "last modification":timestamp, "display name":string, "uri":string}
  T42 = typedef "NI_WebDAV.lvlib/SessionHandle.ctl" = refnum<k1>
  T43 = enum32{"invalid app kind", "Development System", "Run Time System", "Student Edition", "Embedded LabVIEW", "Evaluation", "Custom"}
  T44 = cluster{"App Kind":enum32{"invalid app kind", "Development System", "Run Time System", "Student Edition", "Embedded LabVIEW", "Evaluation", "Custom"}, "This VI":refnum<vi>, "Timeout":i32, "State":T40, "State First Call":bool, "Request Q":refnum<queue>, "FP Data":refnum<class "DecFrame_FP.lvclass">, "Current Time":timestamp, "Start Time":timestamp, "Attempts":i32, "Max Attempts":i32, "Message":string, "RIO IP List":string[], "IP Index":i32, "RIO url":string, "PC Path":path, "Valid RIO Connection":bool, "RIO Folder Found":bool, "Wait Time":dbl, "PC Folder Found":bool, "Current Tab":enum32{"Module Specific", "Azimuth Config", "Drive Config", "Sholder Config", "ExtendFX Config", "Wrist Config", "ExtendProgram Config", "Grabber Config", "Auto PC Config", "Auto Rio Config"}, "PC Azimuth Config":T15, "PC Drive Config":T24, "RIO Azimuth Config":T15, "RIO Drive Config":T24, "PC Config NOT Saved":bool, "WebDAV Ref":T42, "RIO Teams Folder":string, "username":string, "password":string, "PC Module Specific Data":T12, "RIO Module Specific Data":T12, "PC Wrist Config":T36, "RIO Wrist Config":T36, "PC ConeStabber Config":T37, "RIO ConeStabber Config":T37, "PC Extender Config":T34, "RIO Extender Config":T34, "PC Sholder Config":T26, "RIO Sholder Config":T26, "PC Grabber Config":T38, "RIO Grabber Config":T38, "PC file list":string[], "RIO List":T41[]}
  T45 = typedef "ENUM RB_Pos_Quadrant Position.ctl" = enum32{"LFT-TOP", "MID-TOP", "RGT-TOP", "LFT-CTR", "MID-CTR", "RGT-CTR", "LFT-BOT", "MID-BOT", "RGT-BOT"}
  T46 = enum32{"Invalid", "Standard", "Closed", "Hidden", "Minimized", "Maximized"}
  T47 = typedef "DialogType.ctl" = u16
  T48 = typedef "ENUM_State PC File Manager.ctl" = enum16{"<Startup>", "Waiting for Connection", "Waiting for Valid Folder", "Waiting for Instruction", "<Shutdown>"}
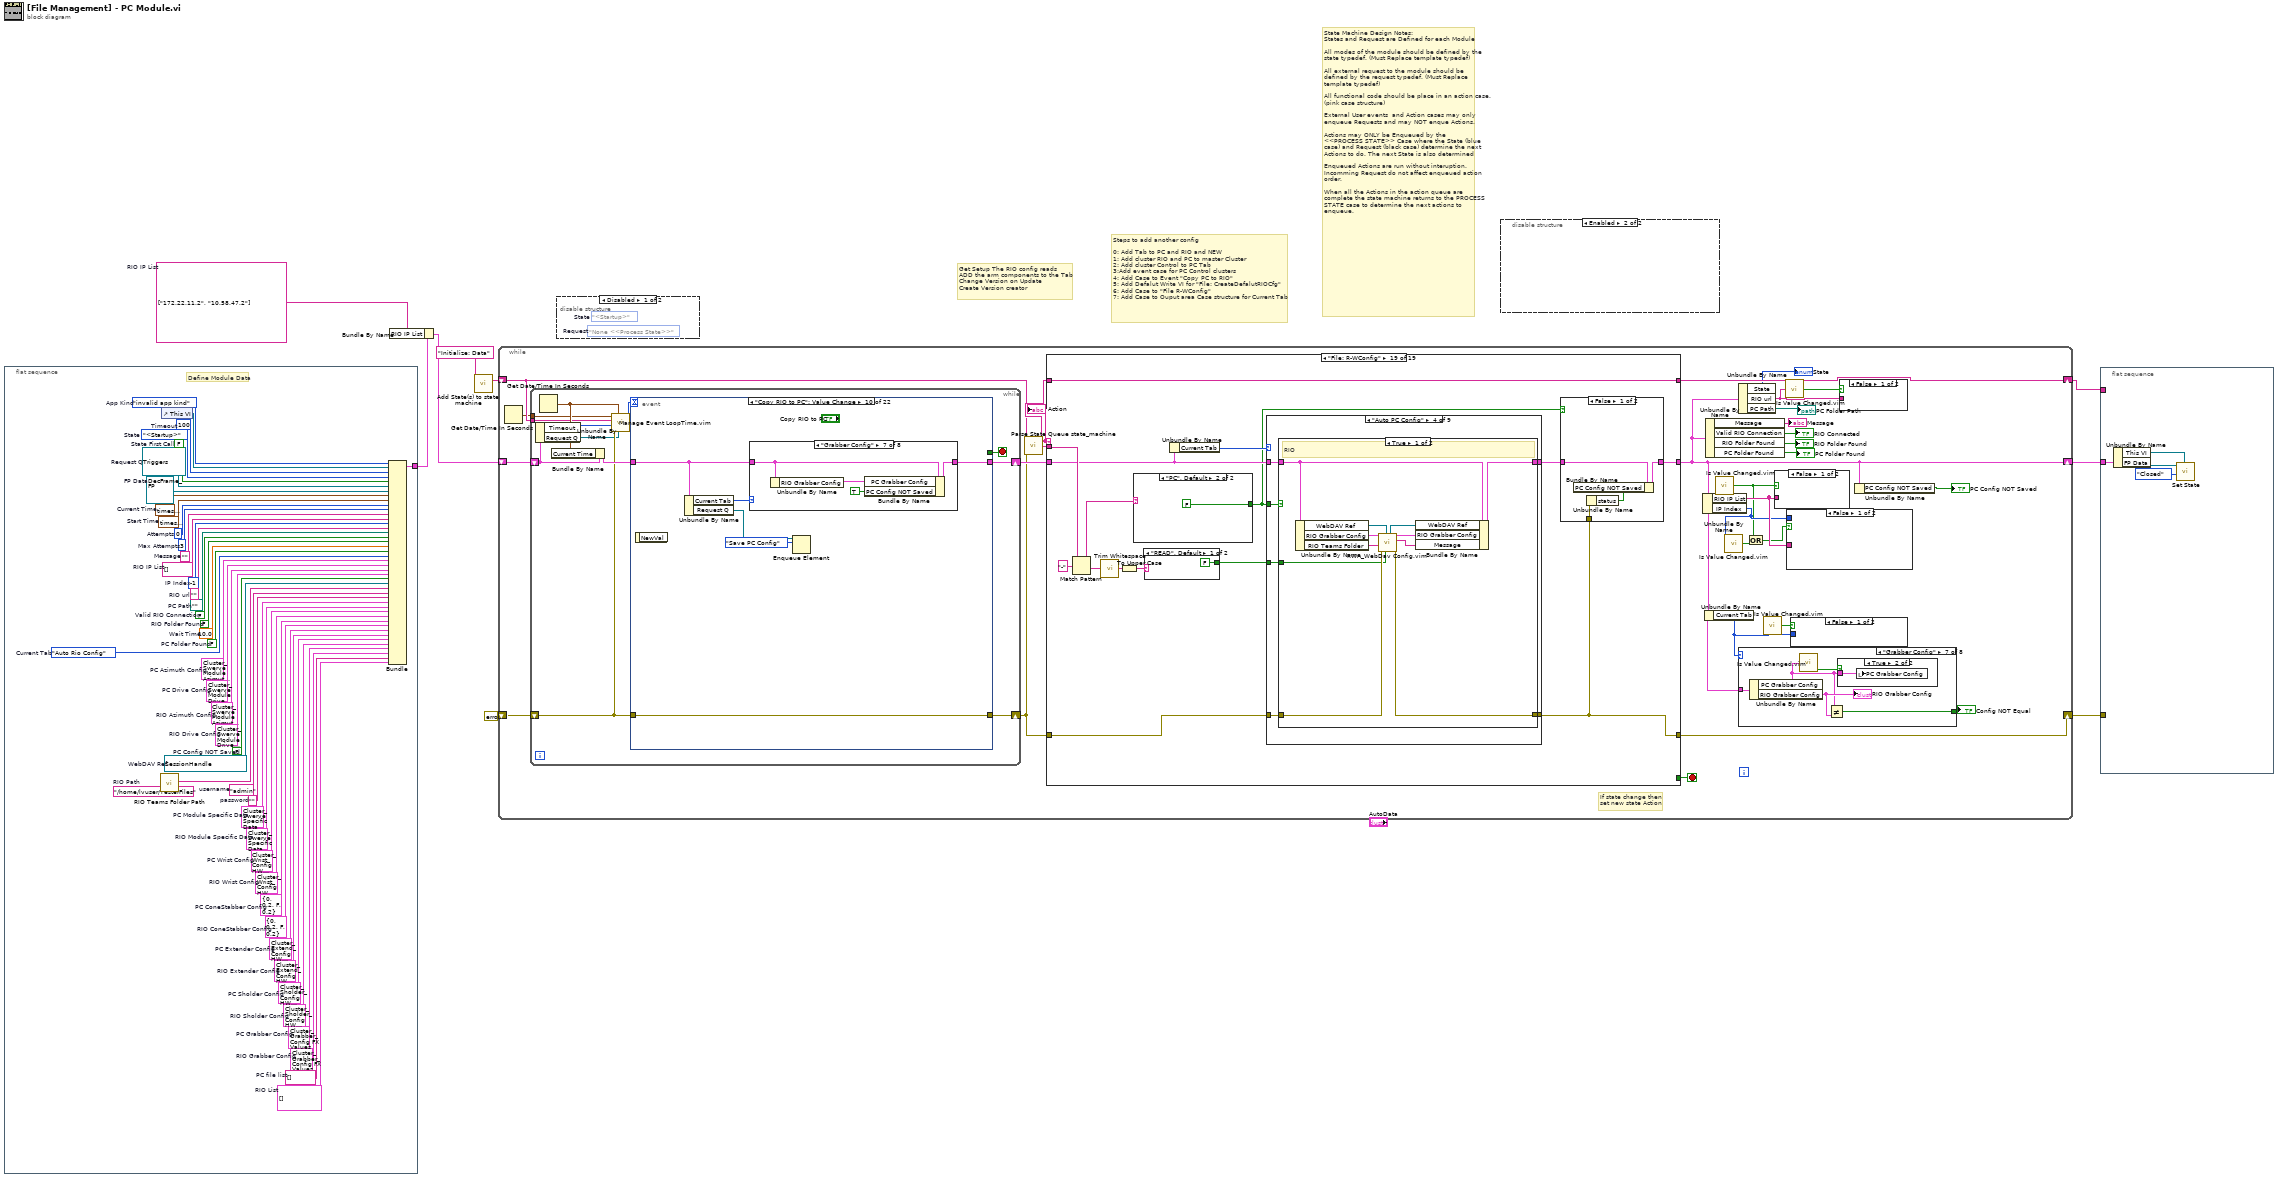
[diagram p0: block diagram]
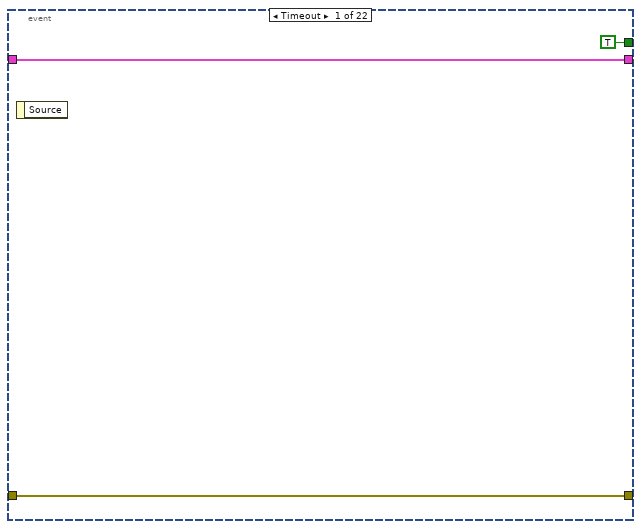
[diagram p2: hidden frame]
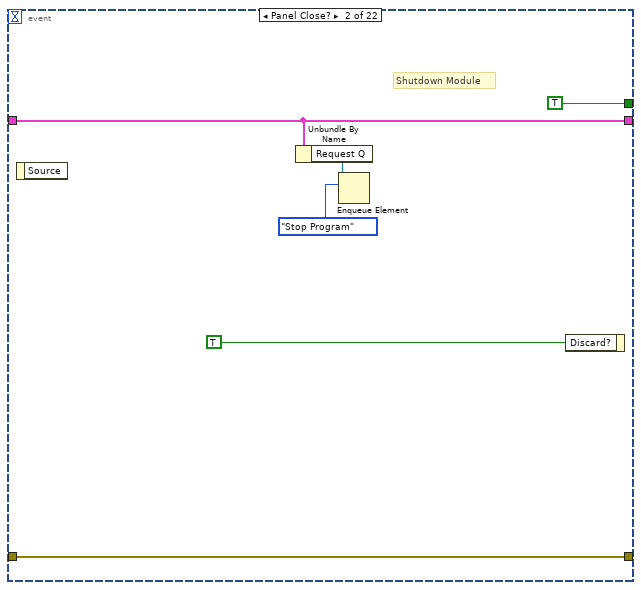
[diagram p3: hidden frame]
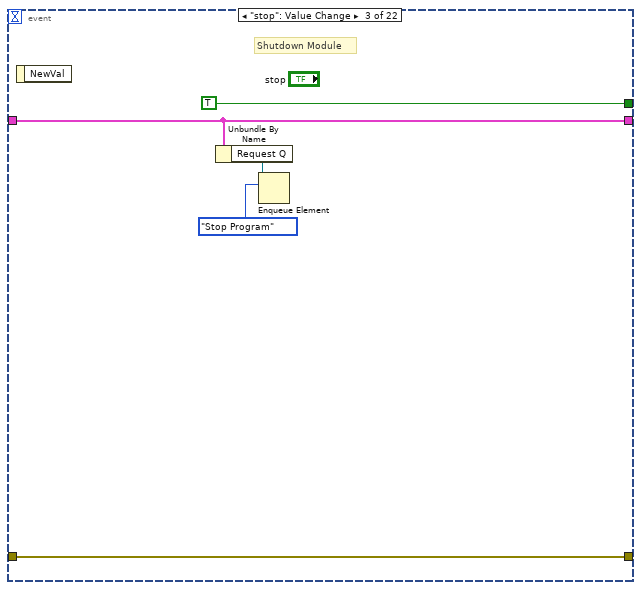
[diagram p4: hidden frame]
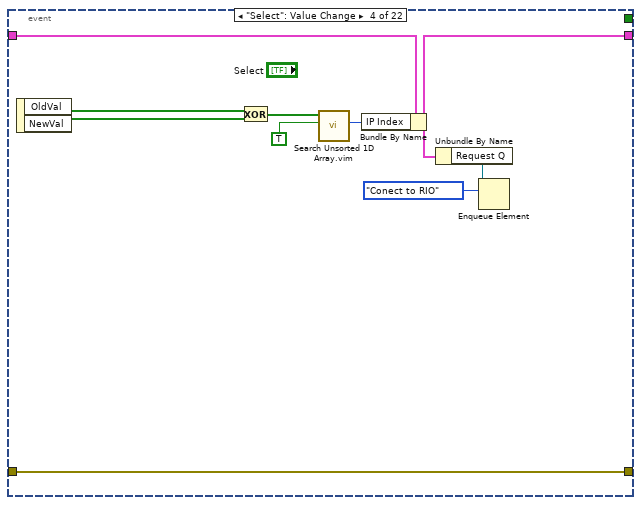
[diagram p5: hidden frame]
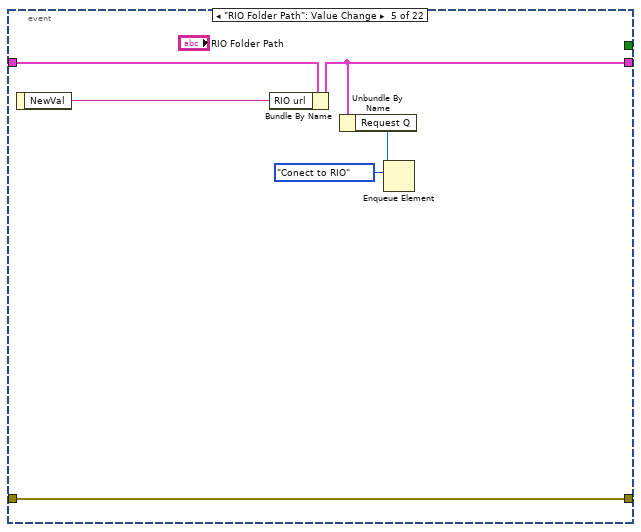
[diagram p6: hidden frame]
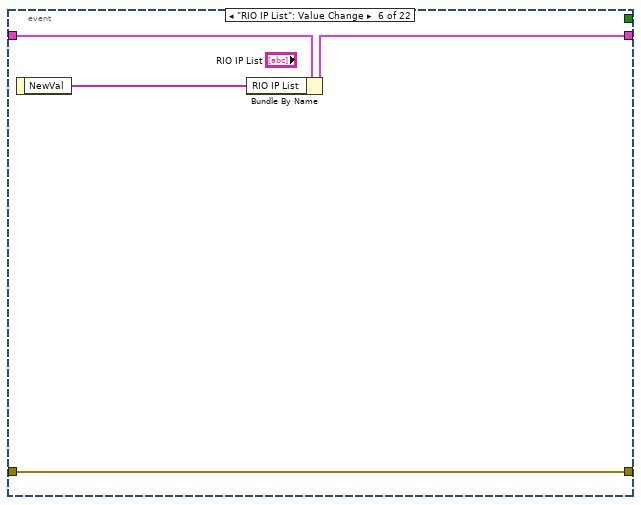
[diagram p7: hidden frame]
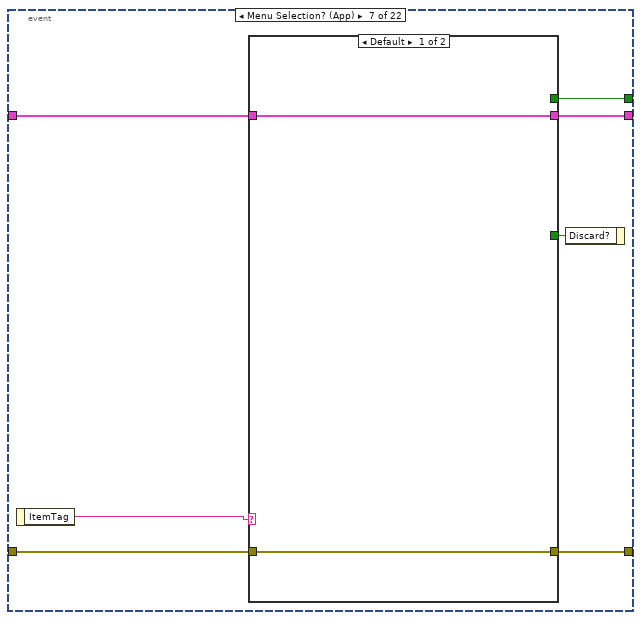
[diagram p8: hidden frame]
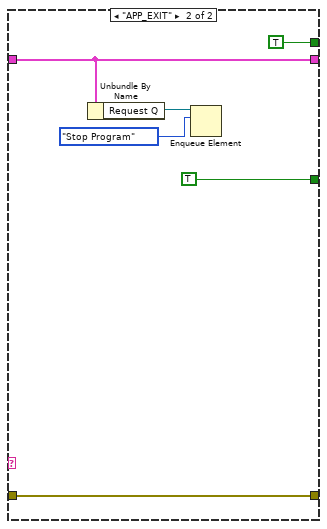
[diagram p9: hidden frame]
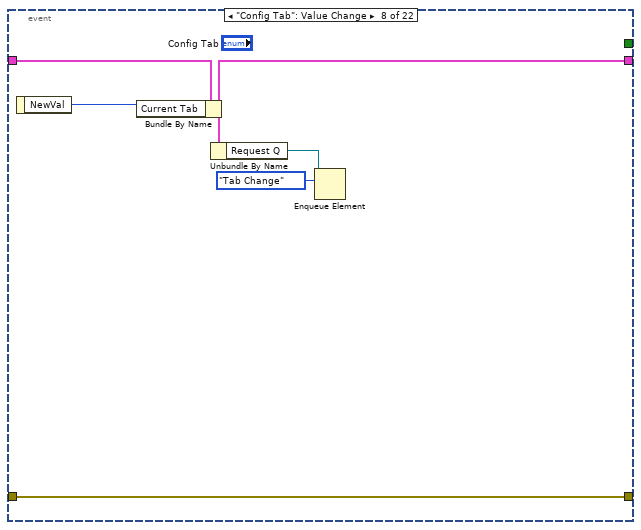
[diagram p10: hidden frame]
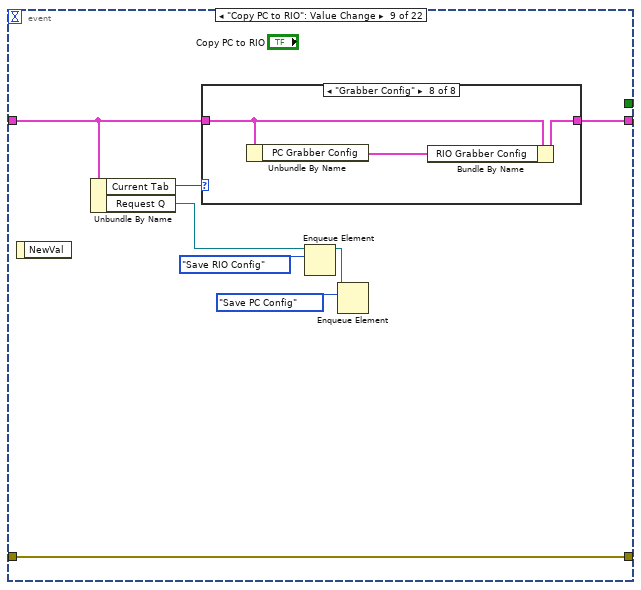
[diagram p11: hidden frame]
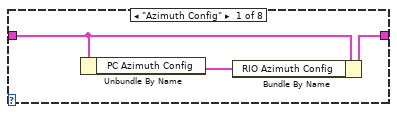
[diagram p12: hidden frame]
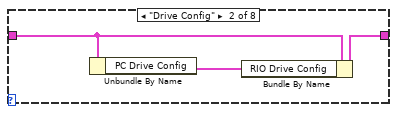
[diagram p13: hidden frame]
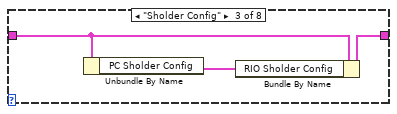
[diagram p14: hidden frame]
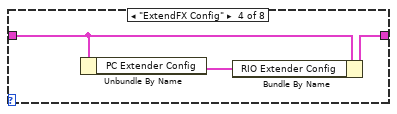
[diagram p15: hidden frame]
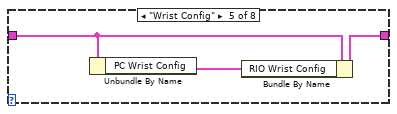
[diagram p16: hidden frame]
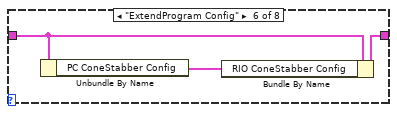
[diagram p17: hidden frame]
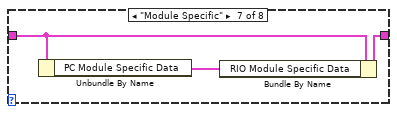
[diagram p18: hidden frame]
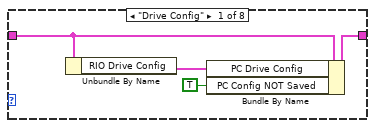
[diagram p19: hidden frame]
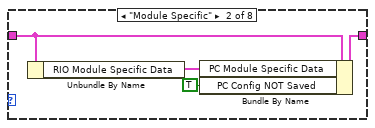
[diagram p20: hidden frame]
diagram:
  w1 = string[] ["172.22.11.2", "10.58.47.2"]  # RIO IP List
  # "Steps to add another config\n\n0: Add Tab to PC and RIO and NEW\n1: Add cluster RIO and PC to master Cluster\n2: Add cluster Control to PC Tab\n3:Add event case for PC Control clusters\n4: Add Case to Event \"Copy PC to RIO\"\n5: Add Defalut Write VI for \"File: CreateDefalutRIOCfg\"\n6: Add Case to \"File R-WConfig\"\n7: Add Case to Ouput area Case structure for Current Tab"
  # "Get Setup The RIO config reads\nADD the arm components to the Tab\nChange Version on Update\nCreate Version creator"
  # "If state change then \nset new state Action"
  # "State Machine Design Notes:\nStates and Request are Defined for each Module\n\nAll modes of the module should be defined by the state typedef. (Must Replace template typedef)\n\nAll external request to the module should be\ndefined by the request typedef. (Must Replace template typedef)\n\nAll functional code should be place in an action case. (pink case structure)\n\nExternal User events  and Action cases may only enqueue Requests and may NOT enque Actions.\n\nActions may ONLY be Enqueued by the\n<<PROCESS STATE>> Case where the State (blue case) and Request (black case) determine the next Actions to do. The next State is also determined\n\nEnqueued Actions are run without interuption.\nIncomming Request do not affect enqueued action order.\n\nWhen all the Actions in the action queue are complete the state machine returns to the PROCESS STATE case to determine the next actions to enqueue."
  n1 = flat-sequence {
    tunnel: [w54] -> w3
    frame #0 {
      w10 = T11."Auto Rio Config"  # Current Tab
      w11 = T41[] []  # RIO List
      w12 = string[] []  # PC file list
      w13 = T38 {"Grabber Ver"=0, "CAN"={"ID"=136, "Bus"=""}, "Output"={"Type"=enum."Counter-Clockwise", "Neutral"=enum."Override to Brake", "Max"={"FWD"=0.0, "REV"=5000.0}, "Min"={"FWD"=0.0, "REV"=0.0}, "OL Ramp Rate (S)"=0.0, "Dead Band"=0.0}, "StatorLimit"={"Enable"=FALSE, "Current Limit"=0.0, "Threshold Current"=0.0, "Threshold Time"=0.0}}  # RIO Grabber Config
      w14 = T38 {"Grabber Ver"=0, "CAN"={"ID"=136, "Bus"=""}, "Output"={"Type"=enum."Counter-Clockwise", "Neutral"=enum."Override to Brake", "Max"={"FWD"=0.0, "REV"=5000.0}, "Min"={"FWD"=0.0, "REV"=0.0}, "OL Ramp Rate (S)"=0.0, "Dead Band"=0.0}, "StatorLimit"={"Enable"=FALSE, "Current Limit"=0.0, "Threshold Current"=0.0, "Threshold Time"=0.0}}  # PC Grabber Config
      w23 = T12 {"SpecificData Ver"=0, "Data"=[{"Motor Pos"=enum."Left-Front", "CAN Bus"="", "Drive ID"=5, "Azimuth ID"=1, "CanCoder ID"=1, "CanCoder Offset"=14.502}, {"Motor Pos"=enum."Right-Front", "CAN Bus"="", "Drive ID"=6, "Azimuth ID"=2, "CanCoder ID"=2, "CanCoder Offset"=166.816}, {"Motor Pos"=enum."Right-Back", "CAN Bus"="", "Drive ID"=7, "Azimuth ID"=3, "CanCoder ID"=3, "CanCoder Offset"=50.273}, {"Motor Pos"=enum."Left-Back", "CAN Bus"="", "Drive ID"=8, "Azimuth ID"=4, "CanCoder ID"=4, "CanCoder Offset"=332.842}]}  # RIO Module Specific Data
      w21 = T36 {"WristHW Ver"=0, "CAN"={"ID"=0, "Bus"=""}, "Output"={"Type"=enum."Counter-Clockwise", "Neutral"=enum."Override to Brake", "Max"={"FWD"=0.0, "REV"=-1.0}, "Min"={"FWD"=0.0, "REV"=0.0}, "OL Ramp Rate (S)"=0.0, "Dead Band"=0.0}, "CL"={"Gains"={"P"=1.0, "I"=0.01, "D"=0.0, "F"=0.0}, "Error Allowed"={"High"=0.0, "Low"=0.0}, "I Zone"={"High"=10000.0, "Low"=-1000.0}, "Max Out"={"FWD"=1.0, "REV"=-1.0}, "Max I Accu"={"High"=10.0, "Low"=-10.0}, "CL Ramp Rate (S)"=0.0}, "MM"={"Cruise Velocity"=5000, "Acceleration"=5000}, "TravelLimits"={"Hard"={"FWD Switch Normal"=enum."Normally Open", "FWD On will Zero Encoder "=FALSE, "REV Switch Normal"=enum."Normally Open", "REV On will Zero Encoder "=FALSE}, "Soft"={"FWD"={"Enable"=FALSE, "Counts"=0}, "REV"={"Enable"=FALSE, "Counts"=0}}}, "Cancoder"={"ID"=0, "CW(t) CCW(f)"=TRUE, "Zero Offset"=0.0}, "CurrentLimit"={"Enable"=FALSE, "Current Limit"=0.0, "Threshold Current"=0.0, "Threshold Time"=0.0}}  # RIO Wrist Config
      w19 = T37 {"ExtendSW Ver"=0, "Home Speed (0-1)"=0.2, "Enable Current Limit On Homing"=FALSE, "At Position Delay(S)"=0.2}  # RIO ConeStabber Config
      w17 = T34 {"ExtendHW Ver"=0, "CAN"={"ID"=0, "Bus"=""}, "Output"={"Type"=enum."Counter-Clockwise", "Neutral"=enum."Override to Brake", "Max"={"FWD"=0.0, "REV"=-1.0}, "Min"={"FWD"=0.0, "REV"=0.0}, "OL Ramp Rate (S)"=0.0, "Dead Band"=0.0}, "CL"={"Gains"={"P"=1.0, "I"=0.01, "D"=0.0, "F"=0.0}, "Error Allowed"={"High"=0.0, "Low"=0.0}, "I Zone"={"High"=10000.0, "Low"=-1000.0}, "Max Out"={"FWD"=1.0, "REV"=-1.0}, "Max I Accu"={"High"=10.0, "Low"=-10.0}, "CL Ramp Rate (S)"=0.0}, "MM"={"Cruise Velocity"=5000, "Acceleration"=5000}, "TravelLimits"={"Hard"={"FWD Switch Normal"=enum."Normally Open", "FWD On will Zero Encoder "=FALSE, "REV Switch Normal"=enum."Normally Open", "REV On will Zero Encoder "=FALSE}, "Soft"={"FWD"={"Enable"=FALSE, "Counts"=0}, "REV"={"Enable"=FALSE, "Counts"=0}}}, "StatorLimit"={"Enable"=FALSE, "Current Limit"=0.0, "Threshold Current"=0.0, "Threshold Time"=0.0}, "Cancoder"={"ID"=0, "CW(t) CCW(f)"=FALSE, "Zero Offset"=0.0}}  # RIO Extender Config
      w15 = T26 {"SholderHW Ver"=0, "CAN"={"ID"=0, "Bus"=""}, "Output"={"Type"=enum."Counter-Clockwise", "Neutral"=enum."Override to Brake", "Max"={"FWD"=0.0, "REV"=-1.0}, "Min"={"FWD"=0.0, "REV"=0.0}, "OL Ramp Rate (S)"=0.0, "Dead Band"=0.0}, "CL"={"Gains"={"P"=1.0, "I"=0.01, "D"=0.0, "F"=0.0}, "Error Allowed"={"High"=0.0, "Low"=0.0}, "I Zone"={"High"=10000.0, "Low"=-1000.0}, "Max Out"={"FWD"=1.0, "REV"=-1.0}, "Max I Accu"={"High"=10.0, "Low"=-10.0}, "CL Ramp Rate (S)"=0.0}, "MM"={"Cruise Velocity"=5000, "Acceleration"=5000}, "TravelLimits"={"Hard"={"FWD Switch Normal"=enum."Normally Open", "FWD On will Zero Encoder "=FALSE, "REV Switch Normal"=enum."Normally Open", "REV On will Zero Encoder "=FALSE}, "Soft"={"FWD"={"Enable"=FALSE, "Counts"=0}, "REV"={"Enable"=FALSE, "Counts"=0}}}, "Cancoder"={"ID"=0, "CW(t) CCW(f)"=TRUE, "Zero Offset"=0.0}}  # RIO Sholder Config
      w24 = T12 {"SpecificData Ver"=0, "Data"=[{"Motor Pos"=enum."Left-Front", "CAN Bus"="", "Drive ID"=5, "Azimuth ID"=1, "CanCoder ID"=1, "CanCoder Offset"=14.502}, {"Motor Pos"=enum."Right-Front", "CAN Bus"="", "Drive ID"=6, "Azimuth ID"=2, "CanCoder ID"=2, "CanCoder Offset"=166.816}, {"Motor Pos"=enum."Right-Back", "CAN Bus"="", "Drive ID"=7, "Azimuth ID"=3, "CanCoder ID"=3, "CanCoder Offset"=50.273}, {"Motor Pos"=enum."Left-Back", "CAN Bus"="", "Drive ID"=8, "Azimuth ID"=4, "CanCoder ID"=4, "CanCoder Offset"=332.842}]}  # PC Module Specific Data
      w22 = T36 {"WristHW Ver"=0, "CAN"={"ID"=0, "Bus"=""}, "Output"={"Type"=enum."Counter-Clockwise", "Neutral"=enum."Override to Brake", "Max"={"FWD"=0.0, "REV"=-1.0}, "Min"={"FWD"=0.0, "REV"=0.0}, "OL Ramp Rate (S)"=0.0, "Dead Band"=0.0}, "CL"={"Gains"={"P"=1.0, "I"=0.01, "D"=0.0, "F"=0.0}, "Error Allowed"={"High"=0.0, "Low"=0.0}, "I Zone"={"High"=10000.0, "Low"=-1000.0}, "Max Out"={"FWD"=1.0, "REV"=-1.0}, "Max I Accu"={"High"=10.0, "Low"=-10.0}, "CL Ramp Rate (S)"=0.0}, "MM"={"Cruise Velocity"=5000, "Acceleration"=5000}, "TravelLimits"={"Hard"={"FWD Switch Normal"=enum."Normally Open", "FWD On will Zero Encoder "=FALSE, "REV Switch Normal"=enum."Normally Open", "REV On will Zero Encoder "=FALSE}, "Soft"={"FWD"={"Enable"=FALSE, "Counts"=0}, "REV"={"Enable"=FALSE, "Counts"=0}}}, "Cancoder"={"ID"=0, "CW(t) CCW(f)"=TRUE, "Zero Offset"=0.0}, "CurrentLimit"={"Enable"=FALSE, "Current Limit"=0.0, "Threshold Current"=0.0, "Threshold Time"=0.0}}  # PC Wrist Config
      w20 = T37 {"ExtendSW Ver"=0, "Home Speed (0-1)"=0.2, "Enable Current Limit On Homing"=FALSE, "At Position Delay(S)"=0.2}  # PC ConeStabber Config
      w18 = T34 {"ExtendHW Ver"=0, "CAN"={"ID"=0, "Bus"=""}, "Output"={"Type"=enum."Counter-Clockwise", "Neutral"=enum."Override to Brake", "Max"={"FWD"=0.0, "REV"=-1.0}, "Min"={"FWD"=0.0, "REV"=0.0}, "OL Ramp Rate (S)"=0.0, "Dead Band"=0.0}, "CL"={"Gains"={"P"=1.0, "I"=0.01, "D"=0.0, "F"=0.0}, "Error Allowed"={"High"=0.0, "Low"=0.0}, "I Zone"={"High"=10000.0, "Low"=-1000.0}, "Max Out"={"FWD"=1.0, "REV"=-1.0}, "Max I Accu"={"High"=10.0, "Low"=-10.0}, "CL Ramp Rate (S)"=0.0}, "MM"={"Cruise Velocity"=5000, "Acceleration"=5000}, "TravelLimits"={"Hard"={"FWD Switch Normal"=enum."Normally Open", "FWD On will Zero Encoder "=FALSE, "REV Switch Normal"=enum."Normally Open", "REV On will Zero Encoder "=FALSE}, "Soft"={"FWD"={"Enable"=FALSE, "Counts"=0}, "REV"={"Enable"=FALSE, "Counts"=0}}}, "StatorLimit"={"Enable"=FALSE, "Current Limit"=0.0, "Threshold Current"=0.0, "Threshold Time"=0.0}, "Cancoder"={"ID"=0, "CW(t) CCW(f)"=FALSE, "Zero Offset"=0.0}}  # PC Extender Config
      w16 = T26 {"SholderHW Ver"=0, "CAN"={"ID"=0, "Bus"=""}, "Output"={"Type"=enum."Counter-Clockwise", "Neutral"=enum."Override to Brake", "Max"={"FWD"=0.0, "REV"=-1.0}, "Min"={"FWD"=0.0, "REV"=0.0}, "OL Ramp Rate (S)"=0.0, "Dead Band"=0.0}, "CL"={"Gains"={"P"=1.0, "I"=0.01, "D"=0.0, "F"=0.0}, "Error Allowed"={"High"=0.0, "Low"=0.0}, "I Zone"={"High"=10000.0, "Low"=-1000.0}, "Max Out"={"FWD"=1.0, "REV"=-1.0}, "Max I Accu"={"High"=10.0, "Low"=-10.0}, "CL Ramp Rate (S)"=0.0}, "MM"={"Cruise Velocity"=5000, "Acceleration"=5000}, "TravelLimits"={"Hard"={"FWD Switch Normal"=enum."Normally Open", "FWD On will Zero Encoder "=FALSE, "REV Switch Normal"=enum."Normally Open", "REV On will Zero Encoder "=FALSE}, "Soft"={"FWD"={"Enable"=FALSE, "Counts"=0}, "REV"={"Enable"=FALSE, "Counts"=0}}}, "Cancoder"={"ID"=0, "CW(t) CCW(f)"=TRUE, "Zero Offset"=0.0}}  # PC Sholder Config
      (unwired) "/home/lvuser/TesterFiles"  # RIO Path
      w26 = ""  # password
      w27 = "admin"  # username
      w28 = T42 refnum items=["Session NI_WebDAV"]  # WebDAV Ref
      w29 = FALSE  # PC Config NOT Saved
      w33 = T15 {"ModuleAzimuth Ver"=0, "Output"={"Type"=enum."Clockwise", "Neutral"=enum."Override to Brake", "Max"={"FWD"=0.0, "REV"=2.0}, "Min"={"FWD"=0.0, "REV"=-1000.0}, "OL Ramp Rate (S)"=0.0, "Dead Band"=0.0}, "CL"={"Gains"={"P"=0.0, "I"=0.0, "D"=20.0, "F"=0.0}, "Error Allowed"={"High"=0.0, "Low"=0.0}, "I Zone"={"High"=0.0, "Low"=0.0}, "Max Out"={"FWD"=20.0, "REV"=0.0}, "Max I Accu"={"High"=1.0, "Low"=-1.0}, "CL Ramp Rate (S)"=0.0}, "MM"={"Cruise Velocity"=0, "Acceleration"=0}}  # PC Azimuth Config
      w32 = T24 {"ModuleDrive Ver"=0, "Output"={"Type"=enum."Counter-Clockwise", "Neutral"=enum."EEPROMSetting", "Max"={"FWD"=0.0, "REV"=0.0}, "Min"={"FWD"=0.0, "REV"=0.0}, "OL Ramp Rate (S)"=0.0, "Dead Band"=0.0}, "CL"={"Gains"={"P"=1.0, "I"=0.01, "D"=0.0, "F"=0.0}, "Error Allowed"={"High"=0.1, "Low"=-0.1}, "I Zone"={"High"=10.0, "Low"=-10.0}, "Max Out"={"FWD"=100.0, "REV"=-100.0}, "Max I Accu"={"High"=0.0, "Low"=0.0}, "CL Ramp Rate (S)"=0.0}, "VoltageComp"={"Enable"=FALSE, "Value"=0.0}}  # PC Drive Config
      w31 = T15 {"ModuleAzimuth Ver"=0, "Output"={"Type"=enum."Clockwise", "Neutral"=enum."Override to Brake", "Max"={"FWD"=0.0, "REV"=2.0}, "Min"={"FWD"=0.0, "REV"=-1000.0}, "OL Ramp Rate (S)"=0.0, "Dead Band"=0.0}, "CL"={"Gains"={"P"=0.0, "I"=0.0, "D"=20.0, "F"=0.0}, "Error Allowed"={"High"=0.0, "Low"=0.0}, "I Zone"={"High"=0.0, "Low"=0.0}, "Max Out"={"FWD"=20.0, "REV"=0.0}, "Max I Accu"={"High"=1.0, "Low"=-1.0}, "CL Ramp Rate (S)"=0.0}, "MM"={"Cruise Velocity"=0, "Acceleration"=0}}  # RIO Azimuth Config
      w30 = T24 {"ModuleDrive Ver"=0, "Output"={"Type"=enum."Counter-Clockwise", "Neutral"=enum."EEPROMSetting", "Max"={"FWD"=0.0, "REV"=0.0}, "Min"={"FWD"=0.0, "REV"=0.0}, "OL Ramp Rate (S)"=0.0, "Dead Band"=0.0}, "CL"={"Gains"={"P"=1.0, "I"=0.01, "D"=0.0, "F"=0.0}, "Error Allowed"={"High"=0.1, "Low"=-0.1}, "I Zone"={"High"=10.0, "Low"=-10.0}, "Max Out"={"FWD"=100.0, "REV"=-100.0}, "Max I Accu"={"High"=0.0, "Low"=0.0}, "CL Ramp Rate (S)"=0.0}, "VoltageComp"={"Enable"=FALSE, "Value"=0.0}}  # RIO Drive Config
      w34 = FALSE  # PC Folder Found
      w35 = 10.0  # Wait Time
      w36 = FALSE  # RIO Folder Found
      w37 = FALSE  # Valid RIO Connection
      w38 = path ""  # PC Path
      w39 = ""  # RIO url
      w40 = -1  # IP Index
      w41 = string[] []  # RIO IP List
      w42 = FALSE  # State First Call
      w43 = ""  # Message
      w44 = 3  # Max Attempts
      w45 = 0  # Attempts
      w46 = timestamp(0 s since 1904-01-01)  # Start Time
      w47 = timestamp(0 s since 1904-01-01)  # Current Time
      w48 = refnum<class "DecFrame_FP.lvclass"> refnum  # FP Data
      w50 = refnum<queue> refnum items=["None <<Process State>>", "Conect to RIO", "SetFP Request", "Stop Program", "Save PC Config", "Save RIO Config", "Read PC Config", "Read RIO Config", "Tab Change"]  # Request Q
      w49 = ENUM_State_PC_File_Manager."<Startup>"  # State
      w52 = T43."invalid app kind"  # App Kind
      w53 = 100  # Timeout
      # "Define Module Data"
      n2 = call "RIO Teams Folder Path.vi"() -> ("RIO Teams Folder"=w25:string)  [unwired: 10 in, 1 out]
      n3 = control-ref of="This VI"() -> (w51:refnum<vi>)
      n4 = Bundle("App Kind"=w52, "This VI"=w51, "Timeout"=w53, "State"=w49, "State First Call"=w42, "Request Q"=w50, "FP Data"=w48, "Current Time"=w47, "Start Time"=w46, "Attempts"=w45, "Max Attempts"=w44, "Message"=w43, "RIO IP List"=w41, "IP Index"=w40, "RIO url"=w39, "PC Path"=w38, "Valid RIO Connection"=w37, "RIO Folder Found"=w36, "Wait Time"=w35, "PC Folder Found"=w34, "Current Tab"=w10, "PC Azimuth Config"=w33, "PC Drive Config"=w32, "RIO Azimuth Config"=w31, "RIO Drive Config"=w30, "PC Config NOT Saved"=w29, "WebDAV Ref"=w28, "RIO Teams Folder"=w25, "username"=w27, "password"=w26, "PC Module Specific Data"=w24, "RIO Module Specific Data"=w23, "PC Wrist Config"=w22, "RIO Wrist Config"=w21, "PC ConeStabber Config"=w20, "RIO ConeStabber Config"=w19, "PC Extender Config"=w18, "RIO Extender Config"=w17, "PC Sholder Config"=w16, "RIO Sholder Config"=w15, "PC Grabber Config"=w14, "RIO Grabber Config"=w13, "PC file list"=w12, "RIO List"=w11) -> (w54:T44)  [unwired: 1 in]
    }
  }
  n5 = Bundle By Name(cluster=w3, "RIO IP List"=w1) -> (w2:T44)
  n6 = call "Add State(s) to state machine.vi"("State(s) in Front (\"\")"="Initialize: Data") -> ("States Out"=w9:string)  [unwired: 14 in]
  n7 = while "JKI - String-Based Queued State Machine (Basic) v1.0" {
    shift-right: [w57] -> w7
    shift-left: w2 -> [w80]
    shift-right: [w73] -> w6
    shift-left: errorcluster {"status"=FALSE, "code"=0, "source"=""} ("Error") -> [w79]
    shift-right: [w82] -> w5
    shift-left: w9 -> [w75]
    stop <- w81 stop-if-true
    n8 = Get Date/Time In Seconds() -> (seconds since 1Jan1904=w71:timestamp)
    n9 = while {
      shift-right: [w95] -> w77
      shift-left: w79 -> [w87]
      shift-right: [w96] -> w78
      shift-left: w80 -> [w93]
      tunnel: w75 -> [w89]
      tunnel: w71 -> [w90]
      stop <- w94 stop-if-true
      n10 = Unbundle By Name(w93) -> ("Timeout"=w88:i32, "Request Q"=w86:refnum<queue>)
      n11 = Get Date/Time In Seconds() -> (seconds since 1Jan1904=w91:timestamp)
      n12 = Bundle By Name(cluster=w93, "Current Time"=w91) -> (w92:T44)
      n13 = call "Manage Event LoopTime.vim"("Request Q"=w86, "Current Time"=w91, "Error"=w87, "Target Time (ms)"=w88, "Action String"=w89, "Start Time"=w90) -> ("Event Time Out"=w85:i32)  [unwired: 5 in]
      n14 = event shown="[9] \"Copy RIO to PC\": Value Change" {
        selector: _ -> [_ _ _ _ _ _ _ _ _ _ _ _ _ _ _ _ _ _ _ _ _ _]
        dyn-events: _ -> [_ _ _ _ _ _ _ _ _ _ _ _ _ _ _ _ _ _ _ _ _ _]
        timeout: w85 -> [_ _ _ _ _ _ _ _ _ _ _ _ _ _ _ _ _ _ _ _ _ _]
        tunnel: w92 -> [w98 w103 w109 w114 w125 w128 w134 w150 w157 w187 w222 w226 w230 w236 w239 w247 w255 w262 w272 w279 w287 w296]
        tunnel: [w99 w105 w110 w120 w126 w130 w136 w151 w159 w189 w225 w229 w233 w237 w245 w253 w261 w270 w278 w286 w294 w302] -> w95
        tunnel: w87 -> [w99 w105 w110 w120 w126 w130 w137 w151 w159 w189 w225 w229 w233 w237 w245 w253 w261 w270 w278 w286 w294 w302]
        tunnel: [w98 w103 w109 w111 w123 w127 w133 w149 w156 w186 w222 w226 w230 w236 w244 w252 w260 w269 w277 w285 w293 w301] -> w96
        tunnel: [TRUE TRUE TRUE _ _ _ w131 _ _ _ _ _ _ _ _ _ _ _ _ _ _ _] -> w94
        event Timeout {
          n15 = event-data() -> ()  [unwired: 1 in, 1 out]
        }
        event Panel Close? {
          # "Shutdown Module"
          n16 = event-data() -> ()  [unwired: 1 in, 1 out]
          n17 = Unbundle By Name(w103) -> ("Request Q"=w101:refnum<queue>)
          n18 = Enqueue Element(queue=w101, element=ENUM_Request_PC_File_Manager."Stop Program") -> ()  [unwired: 2 in, 3 out]
          n19 = event-data("Discard?"=TRUE) -> ()  [unwired: 1 in, 1 out]
        }
        event "stop": Value Change {
          # "Shutdown Module"
          n20 = event-data() -> ()  [unwired: 1 in, 1 out]
          n21 = Unbundle By Name(w109) -> ("Request Q"=w107:refnum<queue>)
          n22 = Enqueue Element(queue=w107, element=ENUM_Request_PC_File_Manager."Stop Program") -> ()  [unwired: 2 in, 3 out]
        }
        event "Select": Value Change {
          n23 = event-data() -> ("OldVal"=w119:bool[], "NewVal"=w118:bool[])  [unwired: 1 in]
          n24 = Exclusive Or(1:w118, 2:w119) -> (0:w117:bool[])
          n25 = call "Search Unsorted 1D Array.vim"("element"=TRUE, "unsorted 1D array"=w117) -> ("index of element"=w115:i32)  [unwired: 9 in]
          n26 = Bundle By Name(cluster=w114, "IP Index"=w115) -> (w111:T44)
          n27 = Unbundle By Name(w111) -> ("Request Q"=w113:refnum<queue>)
          n28 = Enqueue Element(queue=w113, element=ENUM_Request_PC_File_Manager."Conect to RIO") -> ()  [unwired: 2 in, 3 out]
        }
        event "RIO Folder Path": Value Change {
          n29 = event-data() -> ("NewVal"=w124:string)  [unwired: 1 in]
          n30 = Bundle By Name(cluster=w125, "RIO url"=w124) -> (w123:T44)
          n31 = Unbundle By Name(w123) -> ("Request Q"=w122:refnum<queue>)
          n32 = Enqueue Element(queue=w122, element=ENUM_Request_PC_File_Manager."Conect to RIO") -> ()  [unwired: 2 in, 3 out]
        }
        event "RIO IP List": Value Change {
          n33 = event-data() -> ("NewVal"=w129:string[])  [unwired: 1 in]
          n34 = Bundle By Name(cluster=w128, "RIO IP List"=w129) -> (w127:T44)
        }
        event Menu Selection? (App) {
          n35 = event-data() -> ("ItemTag"=w135:string)  [unwired: 1 in]
          n36 = case shown="Default" w135 {
            tunnel: [w139 w145] -> w136
            tunnel: w137 -> [w139 w145]
            tunnel: [_ TRUE] -> w132
            tunnel: w134 -> [w138 w142]
            tunnel: [w138 w142] -> w133
            tunnel: [_ TRUE] -> w131
            frame Default {
            }
            frame "APP_EXIT" {
              n37 = Unbundle By Name(w142) -> ("Request Q"=w141:refnum<queue>)
              n38 = Enqueue Element(queue=w141, element=ENUM_Request_PC_File_Manager."Stop Program") -> ()  [unwired: 2 in, 3 out]
            }
          }
          n39 = event-data("Discard?"=w132) -> ()  [unwired: 1 in, 1 out]
        }
        event "Config Tab": Value Change {
          n40 = event-data() -> ("NewVal"=w146:T11)  [unwired: 1 in]
          n41 = Bundle By Name(cluster=w150, "Current Tab"=w146) -> (w149:T44)
          n42 = Unbundle By Name(w149) -> ("Request Q"=w148:refnum<queue>)
          n43 = Enqueue Element(queue=w148, element=ENUM_Request_PC_File_Manager."Tab Change") -> ()  [unwired: 2 in, 3 out]
        }
        event "Copy PC to RIO": Value Change {
          n44 = event-data() -> ()  [unwired: 1 in, 1 out]
          n45 = Unbundle By Name(w157) -> ("Current Tab"=w158:T11, "Request Q"=w154:refnum<queue>)
          n46 = case shown="\"Grabber Config\"" w158 {
            tunnel: w157 -> [w161 w164 w167 w170 w173 w176 w179 w182]
            tunnel: [w162 w165 w168 w171 w174 w177 w180 w183] -> w156
            frame "Azimuth Config" {
              n47 = Unbundle By Name(w161) -> ("PC Azimuth Config"=w160:T15)
              n48 = Bundle By Name(cluster=w161, "RIO Azimuth Config"=w160) -> (w162:T44)
            }
            frame "Drive Config" {
              n49 = Unbundle By Name(w164) -> ("PC Drive Config"=w163:T24)
              n50 = Bundle By Name(cluster=w164, "RIO Drive Config"=w163) -> (w165:T44)
            }
            frame "Sholder Config" {
              n51 = Unbundle By Name(w167) -> ("PC Sholder Config"=w166:T26)
              n52 = Bundle By Name(cluster=w167, "RIO Sholder Config"=w166) -> (w168:T44)
            }
            frame "ExtendFX Config" {
              n53 = Unbundle By Name(w170) -> ("PC Extender Config"=w169:T34)
              n54 = Bundle By Name(cluster=w170, "RIO Extender Config"=w169) -> (w171:T44)
            }
            frame "Wrist Config" {
              n55 = Unbundle By Name(w173) -> ("PC Wrist Config"=w172:T36)
              n56 = Bundle By Name(cluster=w173, "RIO Wrist Config"=w172) -> (w174:T44)
            }
            frame "ExtendProgram Config" {
              n57 = Unbundle By Name(w176) -> ("PC ConeStabber Config"=w175:T37)
              n58 = Bundle By Name(cluster=w176, "RIO ConeStabber Config"=w175) -> (w177:T44)
            }
            frame "Module Specific" {
              n59 = Unbundle By Name(w179) -> ("PC Module Specific Data"=w178:T12)
              n60 = Bundle By Name(cluster=w179, "RIO Module Specific Data"=w178) -> (w180:T44)
            }
            frame "Grabber Config" {
              n61 = Unbundle By Name(w182) -> ("PC Grabber Config"=w181:T38)
              n62 = Bundle By Name(cluster=w182, "RIO Grabber Config"=w181) -> (w183:T44)
            }
          }
          n63 = Enqueue Element(queue=w154, element=ENUM_Request_PC_File_Manager."Save RIO Config") -> (queue out=w153:refnum<queue>)  [unwired: 2 in, 2 out]
          n64 = Enqueue Element(queue=w153, element=ENUM_Request_PC_File_Manager."Save PC Config") -> ()  [unwired: 2 in, 3 out]
        }
        event "Copy RIO to PC": Value Change {
          n65 = event-data() -> ()  [unwired: 1 in, 1 out]
          n66 = Unbundle By Name(w187) -> ("Current Tab"=w188:T11, "Request Q"=w185:refnum<queue>)
          n67 = case shown="\"Grabber Config\"" w188 {
            tunnel: w187 -> [w192 w196 w200 w204 w208 w212 w216 w220]
            tunnel: [w193 w197 w201 w205 w209 w213 w217 w221] -> w186
            frame "Drive Config" {
              n68 = Unbundle By Name(w192) -> ("RIO Drive Config"=w191:T24)
              n69 = Bundle By Name(cluster=w192, "PC Drive Config"=w191, "PC Config NOT Saved"=TRUE) -> (w193:T44)
            }
            frame "Module Specific" {
              n70 = Unbundle By Name(w196) -> ("RIO Module Specific Data"=w195:T12)
              n71 = Bundle By Name(cluster=w196, "PC Module Specific Data"=w195, "PC Config NOT Saved"=TRUE) -> (w197:T44)
            }
            frame "Azimuth Config" {
              n72 = Unbundle By Name(w200) -> ("RIO Azimuth Config"=w199:T15)
              n73 = Bundle By Name(cluster=w200, "PC Azimuth Config"=w199, "PC Config NOT Saved"=TRUE) -> (w201:T44)
            }
            frame "ExtendFX Config" {
              n74 = Unbundle By Name(w204) -> ("RIO Extender Config"=w203:T34)
              n75 = Bundle By Name(cluster=w204, "PC Extender Config"=w203, "PC Config NOT Saved"=TRUE) -> (w205:T44)
            }
            frame "Wrist Config" {
              n76 = Unbundle By Name(w208) -> ("RIO Wrist Config"=w207:T36)
              n77 = Bundle By Name(cluster=w208, "RIO Wrist Config"=w207, "PC Config NOT Saved"=TRUE) -> (w209:T44)
            }
            frame "ExtendProgram Config" {
              n78 = Unbundle By Name(w212) -> ("RIO ConeStabber Config"=w211:T37)
              n79 = Bundle By Name(cluster=w212, "PC ConeStabber Config"=w211, "PC Config NOT Saved"=TRUE) -> (w213:T44)
            }
            frame "Grabber Config" {
              n80 = Unbundle By Name(w216) -> ("RIO Grabber Config"=w215:T38)
              n81 = Bundle By Name(cluster=w216, "PC Grabber Config"=w215, "PC Config NOT Saved"=TRUE) -> (w217:T44)
            }
            frame "Sholder Config" {
              n82 = Unbundle By Name(w220) -> ("RIO Sholder Config"=w219:T26)
              n83 = Bundle By Name(cluster=w220, "PC Sholder Config"=w219, "PC Config NOT Saved"=TRUE) -> (w221:T44)
            }
          }
          n84 = Enqueue Element(queue=w185, element=ENUM_Request_PC_File_Manager."Save PC Config") -> ()  [unwired: 2 in, 3 out]
        }
        event "Read PC Config": Value Change {
          n85 = event-data() -> ()  [unwired: 1 in, 1 out]
          n86 = Unbundle By Name(w222) -> ("Request Q"=w224:refnum<queue>)
          n87 = Enqueue Element(queue=w224, element=ENUM_Request_PC_File_Manager."Read PC Config") -> ()  [unwired: 2 in, 3 out]
        }
        event "Read RIO Config": Value Change {
          n88 = event-data() -> ()  [unwired: 1 in, 1 out]
          n89 = Unbundle By Name(w226) -> ("Request Q"=w228:refnum<queue>)
          n90 = Enqueue Element(queue=w228, element=ENUM_Request_PC_File_Manager."Read RIO Config") -> ()  [unwired: 2 in, 3 out]
        }
        event "Save PC Config": Value Change {
          n91 = event-data() -> ()  [unwired: 1 in, 1 out]
          n92 = Unbundle By Name(w230) -> ("Request Q"=w232:refnum<queue>)
          n93 = Enqueue Element(queue=w232, element=ENUM_Request_PC_File_Manager."Save PC Config") -> ()  [unwired: 2 in, 3 out]
        }
        event "Save RIO Config": Value Change {
          n94 = event-data() -> ()  [unwired: 1 in, 1 out]
          n95 = Unbundle By Name(w236) -> ("Request Q"=w235:refnum<queue>)
          n96 = Enqueue Element(queue=w235, element=ENUM_Request_PC_File_Manager."Save RIO Config") -> ()  [unwired: 2 in, 3 out]
        }
        event Value Change {
          n97 = event-data() -> ("NewVal"=w243:T24)  [unwired: 1 in, 1 out]
          n98 = Unbundle By Name(w239) -> ("Current Time"=w240:timestamp)
          n99 = call "Date Stamp.vi"("Time"=w240) -> ("U64 Out"=w238:u64)  [unwired: 5 in, 1 out]
          n100 = Bundle By Name(cluster=w243, "ModuleDrive Ver"=w238) -> (w242:T24)
          n101 = Bundle By Name(cluster=w239, "PC Drive Config"=w242, "PC Config NOT Saved"=TRUE) -> (w244:T44)
        }
        event Value Change {
          n102 = event-data() -> ("NewVal"=w251:T38)  [unwired: 1 in, 1 out]
          n103 = Unbundle By Name(w247) -> ("Current Time"=w248:timestamp)
          n104 = call "Date Stamp.vi"("Time"=w248) -> ("U64 Out"=w246:u64)  [unwired: 5 in, 1 out]
          n105 = Bundle By Name(cluster=w251, "Grabber Ver"=w246) -> (w250:T38)
          n106 = Bundle By Name(cluster=w247, "PC Grabber Config"=w250, "PC Config NOT Saved"=TRUE) -> (w252:T44)
        }
        event Value Change {
          n107 = event-data() -> ("NewVal"=w259:T15)  [unwired: 1 in, 1 out]
          n108 = Unbundle By Name(w255) -> ("Current Time"=w256:timestamp)
          n109 = call "Date Stamp.vi"("Time"=w256) -> ("U64 Out"=w254:u64)  [unwired: 5 in, 1 out]
          n110 = Bundle By Name(cluster=w259, "ModuleAzimuth Ver"=w254) -> (w258:T15)
          n111 = Bundle By Name(cluster=w255, "PC Azimuth Config"=w258, "PC Config NOT Saved"=TRUE) -> (w260:T44)
        }
        event Value Change {
          n112 = event-data() -> ("OldVal"=w268:T26, "NewVal"=w265:T26)  [unwired: 1 in]
          n113 = Unbundle By Name(w268) -> ("SholderHW Ver"=w267:u64)
          n114 = Increment(x=w267) -> (x+1=w266:u64)
          n115 = Bundle By Name(cluster=w265, "SholderHW Ver"=w266) -> (w264:T26)
          n116 = Bundle By Name(cluster=w262, "PC Sholder Config"=w264, "PC Config NOT Saved"=TRUE) -> (w269:T44)
        }
        event Value Change {
          n117 = event-data() -> ("NewVal"=w276:T34)  [unwired: 1 in, 1 out]
          n118 = Unbundle By Name(w272) -> ("Current Time"=w273:timestamp)
          n119 = call "Date Stamp.vi"("Time"=w273) -> ("U64 Out"=w271:u64)  [unwired: 5 in, 1 out]
          n120 = Bundle By Name(cluster=w276, "ExtendHW Ver"=w271) -> (w275:T34)
          n121 = Bundle By Name(cluster=w272, "PC Extender Config"=w275, "PC Config NOT Saved"=TRUE) -> (w277:T44)
        }
        event Value Change {
          n122 = event-data() -> ("NewVal"=w284:T36)  [unwired: 1 in, 1 out]
          n123 = Unbundle By Name(w279) -> ("Current Time"=w281:timestamp)
          n124 = call "Date Stamp.vi"("Time"=w281) -> ("U64 Out"=w280:u64)  [unwired: 5 in, 1 out]
          n125 = Bundle By Name(cluster=w284, "WristHW Ver"=w280) -> (w283:T36)
          n126 = Bundle By Name(cluster=w279, "PC Wrist Config"=w283, "PC Config NOT Saved"=TRUE) -> (w285:T44)
        }
        event Value Change {
          n127 = event-data() -> ("NewVal"=w292:T37)  [unwired: 1 in, 1 out]
          n128 = Unbundle By Name(w287) -> ("Current Time"=w289:timestamp)
          n129 = call "Date Stamp.vi"("Time"=w289) -> ("U64 Out"=w288:u64)  [unwired: 5 in, 1 out]
          n130 = Bundle By Name(cluster=w292, "ExtendSW Ver"=w288) -> (w291:T37)
          n131 = Bundle By Name(cluster=w287, "PC ConeStabber Config"=w291, "PC Config NOT Saved"=TRUE) -> (w293:T44)
        }
        event Value Change {
          n132 = event-data() -> ("NewVal"=w300:T12)  [unwired: 1 in, 1 out]
          n133 = Unbundle By Name(w296) -> ("Current Time"=w295:timestamp)
          n134 = call "Date Stamp.vi"("Time"=w295) -> ("U64 Out"=w297:u64)  [unwired: 5 in, 1 out]
          n135 = Bundle By Name(cluster=w300, "SpecificData Ver"=w297) -> (w299:T12)
          n136 = Bundle By Name(cluster=w296, "PC Module Specific Data"=w299, "PC Config NOT Saved"=TRUE) -> (w301:T44)
        }
      }
    }
    n137 = call "Parse State Queue state_machine.vi"("State Queue"=w75, "Error In (no error)"=w77) -> ("Remaining States"=w84:string, "Current State"=w74:string, "Arguments"=w83:string)  [unwired: 11 in]
    "Action" <- w74
    n138 = case shown="\"File: R-WConfig\"" w74 {
      selector: w74 -> [_ _ w818 _ _ _ w854 _ _ _ _ _ _ _ _ _ _ _ _]
      tunnel: w84 -> [w367 w816 w817 w827 w846 w848 w855 w870 w884 w886 w889 w900 w901 w917 w937 w966 w984 w990 w1006]
      tunnel: w83 -> [_ w813 _ _ _ _ w853 _ _ _ _ _ _ _ _ _ _ _ w998]
      tunnel: w78 -> [w368 w810 w820 w830 w841 w851 w861 w871 w881 w888 w890 w895 w902 w907 w933 w958 w982 w987 w996]
      tunnel: [w369 w811 w822 w828 w845 w850 w863 w872 w873 w887 w891 w896 w903 w904 w938 w965 w977 w991 w993] -> w73
      tunnel: w77 -> [w372 w811 w821 w831 w845 w850 w863 w872 w873 w887 w891 w897 w903 w911 w938 w965 w976 w991 w1005]
      tunnel: [w376 w816 w817 w827 w846 w848 w856 w870 w884 w886 w889 w900 w901 w917 w937 w966 w984 w990 w1006] -> w82
      tunnel: [_ _ _ _ _ TRUE _ _ _ _ _ _ _ _ _ _ _ _ _] -> w81
      tunnel: [w363 w812 w820 w829 w841 w851 w861 w871 w885 w888 w890 w894 w902 w908 w934 w957 w983 w989 w994] -> w57
      frame "", "<<PROCESS STATE>>" {
        n139 = Unbundle By Name(w368) -> ("Request Q"=w374:refnum<queue>, "State First Call"=w361:bool, "State"=w371:T40)
        n140 = Dequeue Element(queue=w374, timeout in ms (-1)=0) -> (element=w365:T39)  [unwired: 1 in, 3 out]
        "Next Request" <- w365
        n141 = case shown="\"None <<Process State>>\"" w365 {
          tunnel: w367 -> [w382 _ w713 w728 w740 w756 w774 w792 w806]
          tunnel: [w379 w707 w712 w732 w735 w751 w770 w788 w803] -> w364
          tunnel: [w383 w700 w709 w734 w742 w758 w776 w794 w808] -> w369
          tunnel: w372 -> [w384 w701 w710 w734 w742 w758 w776 w794 w808]
          tunnel: w371 -> [w385 _ w715 _ w738 w754 w773 w791 w807]
          tunnel: [w378 ENUM_State_PC_File_Manager."<Shutdown>" ("State") w711 ENUM_State_PC_File_Manager."Connecting to RIO" ("State") w737 w753 w772 w790 w807] -> w370
          tunnel: w368 -> [w380 w707 w714 w731 w736 w752 w771 w789 w803]
          tunnel: [w381 "" ("Remaining States") w716 w729 w741 w757 w775 w793 w805] -> w366
          tunnel: w361 -> [w377 _ _ _ _ _ _ _ _]
          frame "None <<Process State>>" {
            n142 = case shown="\"Waiting for Valid Folder\"" w385 {
              selector: w385 -> [_ w397 w534 w635 _]
              tunnel: w384 -> [w389 w396 w533 w634 w699]
              tunnel: [w389 w392 w529 w630 w699] -> w383
              tunnel: w382 -> [_ w399 w536 w637 _]
              tunnel: ["UI: FPSet\nInitialize: UI\nFile: BuildPCPath\nWebDAV: Connect" w394 w531 w632 "CleanUp\nExit"] -> w381
              tunnel: w380 -> [w388 w398 w535 w636 w698]
              tunnel: [w388 w393 w530 w631 w698] -> w379
              tunnel: [ENUM_State_PC_File_Manager."Connecting to RIO" ("State") w391 w528 w629 ENUM_State_PC_File_Manager."<Shutdown>" ("State")] -> w378
              tunnel: w377 -> [_ w390 w527 w628 _]
              frame "<Startup>" {
              }
              frame "Connecting to RIO" {
                n143 = while {
                  shift-right: [w403] -> w392
                  shift-left: w396 -> [w404]
                  shift-right: [w405] -> w391
                  shift-left: w397 -> [w406]
                  shift-right: [w401] -> w393
                  shift-left: w398 -> [w402]
                  shift-right: [w409] -> w394
                  shift-left: w399 -> [w410]
                  shift-right: [w407] -> _
                  shift-left: 0 -> [w411]
                  tunnel: w390 -> [w400]
                  stop <- w408 stop-if-true
                  n144 = case shown="1" w411 {
                    selector: w411 -> [w417 w455 w475 _]
                    tunnel: w410 -> [w415 w453 w481 w504]
                    tunnel: [w414 w452 w480 w500] -> w409
                    tunnel: [w413 w449 w478 -1] -> w407
                    tunnel: w406 -> [w421 w458 w477 w495]
                    tunnel: [w422 w459 w476 w496] -> w405
                    tunnel: w404 -> [w420 w457 w474 w498]
                    tunnel: [w419 w456 w474 w497] -> w403
                    tunnel: w402 -> [w418 w451 w482 w503]
                    tunnel: [w416 w454 w479 w501] -> w401
                    tunnel: w400 -> [w412 _ _ _]
                    frame ..0 {
                      # "First Call Check"
                      n145 = case shown="False" w412 {
                        tunnel: [w424 w429] -> w413
                        tunnel: w418 -> [w428 w432]
                        tunnel: [w428 w433] -> w416
                        tunnel: w421 -> [w426 w437]
                        tunnel: [w426 w437] -> w422
                        tunnel: w420 -> [w427 w436]
                        tunnel: [w427 w436] -> w419
                        tunnel: w417 -> [w425 w430]
                        tunnel: w415 -> [w423 w434]
                        tunnel: [w423 w435] -> w414
                        frame False {
                          # "Not First Call for State"
                          n146 = Increment(x=w425) -> (x+1=w424:i32)
                        }
                        frame True {
                          # "First Call for State"
                          n147 = Unbundle By Name(w432) -> ("Valid RIO Connection"=w431:bool)
                          n148 = case shown="False" w431 {
                            tunnel: [w443 w447] -> w435
                            tunnel: w434 -> [w442 w447]
                            tunnel: [w441 w448] -> w433
                            tunnel: w432 -> [w439 w448]
                            tunnel: w430 -> [_ w446]
                            tunnel: [-1 w445] -> w429
                            frame False {
                              n149 = Bundle By Name(cluster=w439, "Valid RIO Connection"=FALSE) -> (w441:T44)
                              n150 = call "Add State(s) to state machine.vi"("State(s) in Front (\"\")"=w442, "State(s) in (\"\")"="WebDAV: Connect") -> ("States Out"=w443:string)  [unwired: 13 in]
                            }
                            frame True {
                              n151 = Increment(x=w446) -> (x+1=w445:i32)
                            }
                          }
                        }
                      }
                    }
                    frame 1 {
                      # "First State Check"
                      n152 = Unbundle By Name(w451) -> ("Valid RIO Connection"=w450:bool)
                      n153 = case shown="True" w450 {
                        tunnel: w451 -> [w465 w466]
                        tunnel: [w465 w468] -> w454
                        tunnel: w458 -> [w462 _]
                        tunnel: [w462 ENUM_State_PC_File_Manager."Waiting for Valid Folder" ("State")] -> w459
                        tunnel: w457 -> [w464 w472]
                        tunnel: [w464 w472] -> w456
                        tunnel: w455 -> [w461 _]
                        tunnel: w453 -> [w463 w471]
                        tunnel: [w463 w471] -> w452
                        tunnel: [w460 -1] -> w449
                        frame False {
                          # "No Connection"
                          n154 = Increment(x=w461) -> (x+1=w460:i32)
                        }
                        frame True {
                          # "Connection"
                          n155 = Bundle By Name(cluster=w466, "Message"="Connected") -> (w468:T44)
                        }
                      }
                    }
                    frame 2 {
                      # "No Connection"
                      n156 = Unbundle By Name(w482) -> ("RIO url"=w473:string)
                      n157 = Empty String/Path?(string/path=w473) -> (empty?=w483:bool)
                      n158 = case shown="True" w483 {
                        tunnel: w482 -> [w484 w491]
                        tunnel: w481 -> [w488 w494]
                        tunnel: [w488 w494] -> w480
                        tunnel: [w484 w492] -> w479
                        tunnel: [w486 -1] -> w478
                        tunnel: w477 -> [w485 w489]
                        tunnel: [w485 w489] -> w476
                        tunnel: w475 -> [w487 _]
                        tunnel: w473 -> [_ _]
                        frame False {
                          # "Path Present"
                          n159 = Increment(x=w487) -> (x+1=w486:i32)
                        }
                        frame True {
                          # "Empty path"
                          n160 = Bundle By Name(cluster=w491, "Message"="No Path Selected") -> (w492:T44)
                        }
                      }
                    }
                    frame 3.. {
                      # "Path Present"
                      n161 = Unbundle By Name(w503) -> ("Current Time"=w502:timestamp, "Start Time"=w508:timestamp, "Wait Time"=w506:dbl)
                      n162 = Subtract(x=w502, y=w508) -> (x-y=w507:dbl)
                      n163 = Greater Or Equal?(x=w507, y=w506) -> (x >= y?=w505:bool)
                      n164 = case shown="False" w505 {
                        tunnel: w504 -> [w516 w526]
                        tunnel: w503 -> [w509 w518]
                        tunnel: w502 -> [_ _]
                        tunnel: [w510 w519] -> w501
                        tunnel: [w516 w525] -> w500
                        tunnel: w498 -> [w515 w522]
                        tunnel: [w515 w522] -> w497
                        tunnel: [w514 w523] -> w496
                        tunnel: w495 -> [w514 w523]
                        frame False {
                          n165 = Unbundle By Name(w509) -> ("RIO url"=w511:string)
                          n166 = Format Into String(format string="Unable to Connect to\n%s" ("Message"), w511) -> (resulting string=w513:string)  [unwired: 2 in, 1 out]
                          n167 = Bundle By Name(cluster=w509, "Message"=w513) -> (w510:T44)
                        }
                        frame True {
                          # "Time Expired"
                          n168 = Unbundle By Name(w518) -> ("RIO url"=w517:string)
                          n169 = Format Into String(format string="Atemting to Connect to\n%s" ("Message"), w517) -> (resulting string=w521:string)  [unwired: 2 in, 1 out]
                          n170 = Bundle By Name(cluster=w518, "Message"=w521) -> (w519:T44)
                          n171 = call "Add State(s) to state machine.vi"("State(s) in Front (\"\")"=w526, "State(s) in (\"\")"="WebDAV: Connect") -> ("States Out"=w525:string)  [unwired: 13 in]
                        }
                      }
                    }
                  }
                  n172 = Less Than 0?(x=w407) -> (x < 0?=w408:bool)
                }
              }
              frame "Waiting for Valid Folder" {
                n173 = while {
                  shift-right: [w540] -> w529
                  shift-left: w533 -> [w541]
                  shift-right: [w542] -> w528
                  shift-left: w534 -> [w543]
                  shift-right: [w538] -> w530
                  shift-left: w535 -> [w539]
                  shift-right: [w546] -> w531
                  shift-left: w536 -> [w547]
                  shift-right: [w544] -> _
                  shift-left: 0 -> [w548]
                  tunnel: w527 -> [w537]
                  stop <- w545 stop-if-true
                  n174 = case shown="1" w548 {
                    selector: w548 -> [w554 w580 _]
                    tunnel: w547 -> [w552 w578 w605]
                    tunnel: [w551 w577 w604] -> w546
                    tunnel: [w550 w574 -1] -> w544
                    tunnel: w543 -> [w558 w583 w608]
                    tunnel: [w559 w584 w607] -> w542
                    tunnel: w541 -> [w557 w582 w609]
                    tunnel: [w556 w581 w606] -> w540
                    tunnel: w539 -> [w555 w576 w603]
                    tunnel: [w553 w579 w602] -> w538
                    tunnel: w537 -> [w549 _ _]
                    frame ..0 {
                      # "First Call Check"
                      n175 = case shown="False" w549 {
                        tunnel: [w560 w566] -> w550
                        tunnel: w555 -> [w565 w570]
                        tunnel: [w565 w571] -> w553
                        tunnel: w558 -> [w563 w573]
                        tunnel: [w563 w573] -> w559
                        tunnel: w557 -> [w564 w572]
                        tunnel: [w564 w572] -> w556
                        tunnel: w554 -> [w561 w567]
                        tunnel: w552 -> [w562 w568]
                        tunnel: [w562 w568] -> w551
                        frame False {
                          # "Not First Call for State"
                          n176 = Increment(x=w561) -> (x+1=w560:i32)
                        }
                        frame True {
                          # "First Call for State"
                          n177 = Increment(x=w567) -> (x+1=w566:i32)
                          n178 = Bundle By Name(cluster=w570, "Attempts"=0) -> (w571:T44)
                        }
                      }
                    }
                    frame 1 {
                      # "First State Check"
                      n179 = Unbundle By Name(w576) -> ("RIO Folder Found"=w575:bool)
                      n180 = case shown="True" w575 {
                        tunnel: w576 -> [w590 w591]
                        tunnel: [w590 w596] -> w579
                        tunnel: w583 -> [w587 _]
                        tunnel: [w587 ENUM_State_PC_File_Manager."Waiting for Instruction" ("State")] -> w584
                        tunnel: w582 -> [w589 w599]
                        tunnel: [w589 w599] -> w581
                        tunnel: w580 -> [w586 _]
                        tunnel: w578 -> [w588 w594]
                        tunnel: [w588 w594] -> w577
                        tunnel: [w585 -1] -> w574
                        frame False {
                          # "First State Check False"
                          n181 = Increment(x=w586) -> (x+1=w585:i32)
                        }
                        frame True {
                          # "First State Check True"
                          n182 = Unbundle By Name(w591) -> ("Request Q"=w593:refnum<queue>)
                          n183 = Enqueue Element(queue=w593, element=ENUM_Request_PC_File_Manager."Tab Change") -> ()  [unwired: 2 in, 3 out]
                          n184 = Bundle By Name(cluster=w591, "Message"="Folder Found") -> (w596:T44)
                        }
                      }
                    }
                    frame 2.. {
                      # "RIO Folder Not found"
                      n185 = Unbundle By Name(w603) -> ("Attempts"=w600:i32, "Max Attempts"=w611:i32)
                      n186 = Less Or Equal?(x=w600, y=w611) -> (x <= y?=w610:bool)
                      n187 = case shown="True" w610 {
                        tunnel: w609 -> [w613 w626]
                        tunnel: w608 -> [w612 w627]
                        tunnel: [w612 w627] -> w607
                        tunnel: [w613 w626] -> w606
                        tunnel: w605 -> [w617 w624]
                        tunnel: [w617 w625] -> w604
                        tunnel: w603 -> [w616 w621]
                        tunnel: [w615 w622] -> w602
                        tunnel: w600 -> [_ w619]
                        frame False {
                          # "Max Attempts exceeded"
                          n188 = Bundle By Name(cluster=w616, "Message"="Unable to Find Teams Folder") -> (w615:T44)
                        }
                        frame True {
                          # "Attempts Allowed"
                          n189 = Increment(x=w619) -> (x+1=w618:i32)
                          n190 = Bundle By Name(cluster=w621, "Attempts"=w618, "Message"="Finding Teams Folder") -> (w622:T44)
                          n191 = call "Add State(s) to state machine.vi"("State(s) in Front (\"\")"=w624, "State(s) in (\"\")"="WebDAV: Find-RIO-Folder") -> ("States Out"=w625:string)  [unwired: 13 in]
                        }
                      }
                    }
                  }
                  n192 = Less Than 0?(x=w544) -> (x < 0?=w545:bool)
                }
              }
              frame "Waiting for Instruction" {
                n193 = while {
                  shift-right: [w641] -> w630
                  shift-left: w634 -> [w642]
                  shift-right: [w643] -> w629
                  shift-left: w635 -> [w644]
                  shift-right: [w639] -> w631
                  shift-left: w636 -> [w640]
                  shift-right: [w647] -> w632
                  shift-left: w637 -> [w648]
                  shift-right: [w645] -> _
                  shift-left: 0 -> [w649]
                  tunnel: w628 -> [w638]
                  stop <- w646 stop-if-true
                  n194 = case shown="1.." w649 {
                    selector: w649 -> [w658 w682]
                    tunnel: w648 -> [w656 w680]
                    tunnel: [w655 w679] -> w647
                    tunnel: [w654 -1] -> w645
                    tunnel: w644 -> [w661 w685]
                    tunnel: [w662 w686] -> w643
                    tunnel: w642 -> [w660 w684]
                    tunnel: [w659 w683] -> w641
                    tunnel: w640 -> [w653 w678]
                    tunnel: [w657 w681] -> w639
                    tunnel: w638 -> [w650 _]
                    frame ..0 {
                      # "First Call Check"
                      n195 = Unbundle By Name(w653) -> ("Valid RIO Connection"=w652:bool)
                      n196 = And(x=w652, y=w650) -> (x .and. y?=w651:bool)
                      n197 = case shown="False" w651 {
                        tunnel: [w663 -1] -> w654
                        tunnel: w653 -> [w668 w675]
                        tunnel: [w668 w675] -> w657
                        tunnel: w661 -> [w666 w674]
                        tunnel: [w666 w674] -> w662
                        tunnel: w660 -> [w667 w673]
                        tunnel: [w667 w673] -> w659
                        tunnel: w658 -> [w664 _]
                        tunnel: w656 -> [w665 w669]
                        tunnel: [w665 w670] -> w655
                        frame False {
                          # "Not First Call for State"
                          n198 = Increment(x=w664) -> (x+1=w663:i32)
                        }
                        frame True {
                          # "First Call for State"
                          n199 = call "Add State(s) to state machine.vi"("State(s) in Front (\"\")"=w669, "State(s) at Back (\"\")"="File: R-WConfig>>RIO-READ\nFile: R-WConfig>>PC-READ" ("State(s) at Back (\"\")")) -> ("States Out"=w670:string)  [unwired: 13 in]
                        }
                      }
                    }
                    frame 1.. {
                      # "First State Check"
                      n200 = Unbundle By Name(w678) -> ("Valid RIO Connection"=w677:bool)
                      n201 = case shown="True" w677 {
                        tunnel: w678 -> [w690 w695]
                        tunnel: [w690 w695] -> w681
                        tunnel: w685 -> [_ w692]
                        tunnel: [ENUM_State_PC_File_Manager."Connecting to RIO" ("State") w692] -> w686
                        tunnel: w684 -> [w689 w694]
                        tunnel: [w689 w694] -> w683
                        tunnel: w682 -> [_ w691]
                        tunnel: w680 -> [w688 w693]
                        tunnel: [w688 w693] -> w679
                        frame False {
                          # "First State Check False"
                        }
                        frame True {
                          # "First State Check True"
                          n202 = Increment(x=w691) -> ()  [unwired: 1 out]
                        }
                      }
                    }
                  }
                  n203 = Less Than 0?(x=w645) -> (x < 0?=w646:bool)
                }
              }
              frame "<Shutdown>" {
              }
            }
          }
          frame "Stop Program" {
            n204 = Unbundle By Name(w707) -> ("Request Q"=w704:refnum<queue>)
            n205 = Flush Queue(queue=w704, error in (no error)=w701) -> (queue out=w703:refnum<queue>, error out=w702:errorcluster)  [unwired: 1 out]
            n206 = Enqueue Element(queue=w703, element=ENUM_Request_PC_File_Manager."None <<Process State>>", error in (no error)=w702) -> (error out=w700:errorcluster)  [unwired: 1 in, 2 out]
          }
          frame "SetFP Request" {
            n207 = case shown="Default" w715 {
              selector: w715 -> [w717 w722]
              tunnel: [w719 w725] -> w716
              tunnel: w714 -> [w718 w723]
              tunnel: w713 -> [w719 w726]
              tunnel: [w718 w723] -> w712
              tunnel: [w717 w722] -> w711
              tunnel: w710 -> [w720 w721]
              tunnel: [w720 w721] -> w709
              frame "<Shutdown>" {
              }
              frame Default {
                n208 = call "Add State(s) to state machine.vi"("State(s) in (\"\")"=w726, "State(s) at Back (\"\")"="UI: FPSet") -> ("States Out"=w725:string)  [unwired: 13 in]
              }
            }
          }
          frame "Conect to RIO" {
            n209 = Bundle By Name(cluster=w731, "Valid RIO Connection"=FALSE) -> (w732:T44)
            n210 = call "Add State(s) to state machine.vi"("State(s) in Front (\"\")"=w728, "State(s) in (\"\")"="WebDAV: Connect" ("State(s) in (\"\")")) -> ("States Out"=w729:string)  [unwired: 13 in]
          }
          frame "Save PC Config" {
            n211 = Unbundle By Name(w736) -> ("PC Folder Found"=w739:bool)
            n212 = case shown="True" w739 {
              tunnel: [w745 w750] -> w741
              tunnel: w740 -> [w745 w749]
              tunnel: w738 -> [_ w746]
              tunnel: [ENUM_State_PC_File_Manager."<Startup>" ("State") w746] -> w737
              tunnel: w736 -> [w744 w747]
              tunnel: [w744 w747] -> w735
              frame False {
                # "Folder invalid"
              }
              frame True {
                # "Folder valid"
                n213 = call "Add State(s) to state machine.vi"("State(s) in Front (\"\")"=w749, "State(s) in (\"\")"="File: R-WConfig>>PC-SAVE\nFile: R-WConfig>>PC-READ" ("State(s) in (\"\")")) -> ("States Out"=w750:string)  [unwired: 13 in]
              }
            }
          }
          frame "Read PC Config" {
            n214 = Unbundle By Name(w752) -> ("PC Folder Found"=w755:bool)
            n215 = case shown="True" w755 {
              tunnel: [w761 w766] -> w757
              tunnel: w756 -> [w761 w765]
              tunnel: w754 -> [_ w762]
              tunnel: [ENUM_State_PC_File_Manager."<Startup>" ("State") w762] -> w753
              tunnel: w752 -> [w760 w763]
              tunnel: [w760 w763] -> w751
              frame False {
                # "Folder invalid"
              }
              frame True {
                # "Folder valid"
                n216 = call "Add State(s) to state machine.vi"("State(s) in Front (\"\")"=w765, "State(s) in (\"\")"="File: R-WConfig>>PC-READ" ("State(s) in (\"\")")) -> ("States Out"=w766:string)  [unwired: 13 in]
              }
            }
          }
          frame "Save RIO Config" {
            n217 = Unbundle By Name(w771) -> ("Valid RIO Connection"=w769:bool, "RIO Folder Found"=w768:bool)
            n218 = And(x=w769, y=w768) -> (x .and. y?=w767:bool)
            n219 = case shown="True" w767 {
              tunnel: [w777 w784] -> w775
              tunnel: w774 -> [w777 w783]
              tunnel: w773 -> [_ w780]
              tunnel: [ENUM_State_PC_File_Manager."Connecting to RIO" ("State") w780] -> w772
              tunnel: w771 -> [w779 w781]
              tunnel: [w779 w781] -> w770
              frame False {
                # "Folder invalid"
              }
              frame True {
                # "Folder valid"
                n220 = call "Add State(s) to state machine.vi"("State(s) in Front (\"\")"=w783, "State(s) in (\"\")"="File: R-WConfig>>RIO-SAVE\nFile: R-WConfig>>RIO-READ" ("State(s) in (\"\")")) -> ("States Out"=w784:string)  [unwired: 13 in]
              }
            }
          }
          frame "Read RIO Config" {
            n221 = Unbundle By Name(w789) -> ("Valid RIO Connection"=w787:bool, "RIO Folder Found"=w786:bool)
            n222 = And(x=w787, y=w786) -> (x .and. y?=w785:bool)
            n223 = case shown="True" w785 {
              tunnel: [w795 w802] -> w793
              tunnel: w792 -> [w795 w801]
              tunnel: w791 -> [_ w798]
              tunnel: [ENUM_State_PC_File_Manager."Connecting to RIO" ("State") w798] -> w790
              tunnel: w789 -> [w797 w799]
              tunnel: [w797 w799] -> w788
              frame False {
                # "Folder invalid"
              }
              frame True {
                # "Folder valid"
                n224 = call "Add State(s) to state machine.vi"("State(s) in Front (\"\")"=w801, "State(s) in (\"\")"="File: R-WConfig>>RIO-READ" ("State(s) in (\"\")")) -> ("States Out"=w802:string)  [unwired: 13 in]
              }
            }
          }
          frame "Tab Change" {
            n225 = call "Add State(s) to state machine.vi"("State(s) in (\"\")"=w806, "State(s) at Back (\"\")"="File: R-WConfig>>RIO-READ\nFile: R-WConfig>>PC-READ" ("State(s) at Back (\"\")")) -> ("States Out"=w805:string)  [unwired: 13 in]
          }
        }
        n226 = Bundle By Name(cluster=w364, "State First Call"=FALSE) -> (w363:T44)
        n227 = call "Build State Change Action.vim"("Current State"=w371, "Target State"=w370) -> ("Action String Out"=w375:string)  [unwired: 3 in]
        n228 = call "Add State(s) to state machine.vi"("State(s) in (\"\")"=w366, "State(s) at Back (\"\")"=w375) -> ("States Out"=w376:string)  [unwired: 13 in]
      }
      frame "State: Change" {
        n229 = Scan From String(input string=w813, default 1=ENUM_State_PC_File_Manager."<Startup>" ("State")) -> (output 1=w814:T40)  [unwired: 3 in, 3 out]
        n230 = Bundle By Name(cluster=w810, "State"=w814, "State First Call"=TRUE) -> (w812:T44)
      }
      frame Default {
        w825 = 42 items=["No error", "Argument error", "Memory is full", "Out of zone", "End of file", "File already open", "Generic file I/O error", "File not found", "File permission error", "Disk is full", "Duplicate path", "Too many files open", "System feature not enabled", "Resource file not found", "Cannot add resource", "Resource not found", "Image not found", "Image memory error", "Pen does not exist", "Config type invalid", "Config token not found", "Config parse error", "Config memory error", "Bad external code format", "Bad external code offset", "External code not present", "Null window", "Destroy window error", "Null menu", "Print aborted", "Bad print record", "Print driver error", "Windows error during printing", "Memory error during printing", "Print dialog error", "Generic print error", "Invalid device refnum", "Device not found", "Device parameter error", "Device unit error", "Cannot open device", "Device call aborted", "Generic error", "Cancelled by user", "Object ID too low", "Object ID too high", "Object not in heap", "Unknown heap", "Unknown object (invalid DefProc)", "Unknown object (DefProc not in table)", "Message out of range", "Invalid (null) method", "Unknown message", "Manager call not supported", "Bad address", "Network operation in progress", "Network operation timed out", "Connection is busy", "Network attribute not supported", "Network error", "Address in use", "System out of memory", "Connection aborted", "Connection refused", "Not connected", "Already connected", "Connection closed", "Initialization error (interapplication manager)", "Bad occurrence", "Wait on unbound occurrence handler", "Occurrence queue overflow", "Datalog type conflict", "Unused", "Unrecognized type (interapplication manager)", "Memory corrupt", "Failed to make temporary DLL", "Old CIN version", "Drag socket not found", "Failed to load drop-object", "Failed to register OLE object", "Failed to release OLE object", "Format specifier type mismatch", "Unknown format specifier", "Too few format specifiers", "Too many format specifiers", "Scan failed", "Newer CIN version", "Error converting to variant", "Runtime menu error", "Password tampered", "Variant attribute not found", "Incompatible variant data type", "Event data is not available", "Event Store is not present", "Occurrence is not found", "Event Queue is not created", "Event info is not available", "Refnum passed is NULL", "Error retrieving Class GUID", "Error retrieving CoClass GUID", "Error retrieving TypeLib GUID.", "Bad built application magic bytes.", "Specific driver is different from the specific driver associated with the Logical Name.", "There is no session opened to the class driver.", "Max Error", "MAX - Error with config objects", "MAX - Error loading configuration", "MAX - Group not supported"]
        n231 = Format Into String(format string="Unable to process Action\nNo Action Case is defined for\n%s" ("message"), error in=w821, w818) -> (resulting string=w824:string, error out=w823:errorcluster)  [unwired: 1 in]
        n232 = call <vilib>:"Error Cluster From Error Code.vi"("show call chain? (False)"=TRUE, "error in (no error)"=w823, "error message (\"\")"=w824, "error code (0)"=w825) -> ("error out"=w822:errorcluster)  [unwired: 5 in]
      }
      frame "Error Handler" {
        n233 = case shown="False" FALSE {
          tunnel: w831 -> [w837 _]
          tunnel: [w836 w839] -> w829
          tunnel: w830 -> [w836 w839]
          tunnel: [errorcluster {"status"=FALSE, "code"=0, "source"=""} ("error out") errorcluster {"status"=FALSE, "code"=0, "source"=""} ("error out")] -> w828
          frame False {
            w833 = T47 2 items=["no dialog", "OK message", "continue or stop message", "OK message + warnings", "continue/stop + warnings"] ("type of dialog (OK msg:1)")
            # "Display error"
            n234 = call <vilib>:"General Error Handler.vi"("type of dialog (OK msg:1)"=w833, "error in (no error)"=w837) -> ("error out"=w834:errorcluster)  [unwired: 9 in, 4 out]
            n235 = flat-sequence {
              tunnel: w834 -> [_]
              frame #0 {
                n236 = Wait (ms)(milliseconds to wait=u32 2000) -> ()  [unwired: 1 out]
              }
            }
          }
          frame True {
            # "Clear error"
          }
        }
      }
      frame "CleanUp" {
        # "Destroy and open refs"
        n237 = Unbundle By Name(w841) -> ("This VI"=w847:refnum<vi>, "Request Q"=w843:refnum<queue>)
        n238 = Close Reference(reference=w847) -> (error out=w844:errorcluster)  [unwired: 1 in]
        n239 = Release Queue(queue=w843) -> (error out=w842:errorcluster)  [unwired: 2 in, 2 out]
        n240 = call <vilib>:"Clear Errors.vi"("error in (no error)"=w844) -> ()  [unwired: 5 in, 2 out]
        n241 = call <vilib>:"Clear Errors.vi"("error in (no error)"=w842) -> ()  [unwired: 5 in, 2 out]
      }
      frame "Exit" {
      }
      frame "Wait" {
        n242 = Fract/Exp String To Number(string=w853, default (0 dbl)=0.0 ("default (0 DBL)")) -> (number=w857:dbl)  [unwired: 2 in, 1 out]
        n243 = Unbundle By Name(w861) -> ("Current Time"=w860:timestamp, "Start Time"=w859:timestamp)
        n244 = Subtract(x=w860, y=w859) -> (x-y=w858:dbl)
        n245 = Greater Or Equal?(x=w858, y=w857) -> (x >= y?=w852:bool)
        n246 = case shown="False" w852 {
          tunnel: [w868 w869] -> w856
          tunnel: w855 -> [w865 w869]
          tunnel: w854 -> [w867 _]
          tunnel: w853 -> [w866 _]
          frame False {
            n247 = call "Build State String with Arguments state_machine.vi"("Arguments (\"\")"=w866, "State"=w867) -> ("State with Arguments"=w864:string)  [unwired: 4 in]
            n248 = call "Add State(s) to state machine.vi"("State(s) in Front (\"\")"=w864, "State(s) in (\"\")"=w865) -> ("States Out"=w868:string)  [unwired: 13 in]
          }
          frame True {
          }
        }
      }
      frame "---------- Initialize ----------" {
      }
      frame "Initialize: Data" {
        w874 = i16 -2  # Border Spacing
        w878 = 0  # Decoration Index
        w879 = u16 0  # Monitor #
        # "INI Data"
        n249 = Unbundle By Name(w881) -> ("FP Data"=w880:refnum<class "DecFrame_FP.lvclass">)
        n250 = property class="App"() -> ("App.Kind"=w877:T43)  [unwired: 2 in, 2 out]
        n251 = call-dynamic "Setup DecFrame Data.vi"("Border Spacing"=w874, "Monitor Select"=w879, "FPLocation"=ENUM_RB_Pos_Quadrant_Position."LFT-TOP", "Decoration Index"=w878, "FP"=w880) -> ("FP Out"=w876:refnum<class "DecFrame_FP.lvclass">)  [unwired: 5 in, 1 out]
        n252 = Obtain Queue(element data type=ENUM_Request_PC_File_Manager."None <<Process State>>" ("Triggers")) -> (queue out=w883:refnum<queue>)  [unwired: 4 in, 2 out]
        n253 = Bundle By Name(cluster=w881, "FP Data"=w876, "App Kind"=w877, "Request Q"=w883) -> (w885:T44)
      }
      frame "Initialize: UI" {
        # "Setup UI indicators and controls"
      }
      frame "---------- UI ----------" {
      }
      frame "UI: FPSet" {
        # "Set FP"
        n254 = Unbundle By Name(w895) -> ("This VI"=w899:refnum<vi>, "FP Data"=w898:refnum<class "DecFrame_FP.lvclass">)
        n255 = call-dynamic "Set State.vi"("VI Ref"=w899, "Error"=w897, "State"=T46."Standard", "FP"=w898) -> ("Error Out"=w896:errorcluster, "FP Out"=w893:refnum<class "DecFrame_FP.lvclass">)  [unwired: 5 in, 1 out]
        n256 = Bundle By Name(cluster=w895, "FP Data"=w893) -> (w894:T44)
      }
      frame "---------- File ----------" {
      }
      frame "File: BuildPCPath" {
        n257 = Current VI's Path() -> (path=w916:path)
        n258 = Strip Path(path=w916) -> (stripped path=w915:path)  [unwired: 1 out]
        n259 = Strip Path(path=w915) -> (stripped path=w914:path)  [unwired: 1 out]
        n260 = Build Path(base path=w914, name or relative path="Team Files") -> (appended path=w912:path)
        n261 = call <vilib>:"Check if File or Folder Exists.vi"("error in (no error)"=w911, "path"=w912) -> ("error out"=w904:errorcluster, "file or folder exists?"=w910:bool, "dup path"=w909:path)  [unwired: 7 in]
        n262 = case shown="False" w910 {
          selector: w910 -> [_ w923]
          tunnel: w909 -> [w921 w922]
          tunnel: [w919 w923] -> w905
          tunnel: [w918 w922] -> w906
          frame False {
            n263 = Create Folder(path (use dialog)=w921) -> (created path=w920:path)  [unwired: 2 in, 2 out]
            n264 = call <vilib>:"Check if File or Folder Exists.vi"("path"=w920) -> ("file or folder exists?"=w919:bool, "dup path"=w918:path)  [unwired: 8 in, 1 out]
          }
          frame True {
          }
        }
        n265 = Bundle By Name(cluster=w907, "PC Path"=w906, "PC Folder Found"=w905) -> (w908:T44)
      }
      frame "WebDAV: Connect" {
        w925 = FALSE ("PC Path Found")
        n266 = Unbundle By Name(w933) -> ("password"=w930:string, "username"=w929:string, "RIO IP List"=w935:string[], "IP Index"=w936:i32, "WebDAV Ref"=w927:T42)
        n267 = call <vilib>:"Close Session.vi"("session handle"=w927) -> ("error out"=w926:errorcluster)  [unwired: 14 in]
        n268 = case shown="0.." w936 {
          selector: w936 -> [_ w955]
          tunnel: w935 -> [_ w956]
          tunnel: ["" w942] -> w932
          tunnel: [w940 w947] -> w931
          tunnel: w930 -> [_ w952]
          tunnel: w929 -> [_ w951]
          tunnel: [FALSE ("Valid RIO Connection") w944] -> w928
          tunnel: w926 -> [_ _]
          tunnel: [_ w943] -> w924
          frame ..-1 {
            w940 = T42 refnum items=["Session NI_WebDAV"] ("session handle out")
          }
          frame 0.. {
            n269 = Index Array(array=w956, index=w955) -> (element=w954:string)
            n270 = Format Into String(format string="http://%s/files", w954) -> (resulting string=w942:string)  [unwired: 2 in, 1 out]
            n271 = call <vilib>:"Open Session.vi"("host uri prefix"=w942, "username"=w951, "password"=w952, "timeout ms"=10000, "verify server?"=TRUE) -> ("session handle out"=w948:T42, "error out"=w946:errorcluster)  [unwired: 9 in]
            n272 = call <vilib>:"Directory Listing.vi"("session handle"=w948, "relative uri"=w942, "error in (no error)"=w946) -> ("session handle out"=w947:T42, "file list"=w943:T41[], "error out"=w945:errorcluster)  [unwired: 9 in, 1 out]
            n273 = Not(x=w945) -> (.not. x?=w944:bool)
          }
        }
        n274 = Bundle By Name(cluster=w933, "RIO url"=w932, "WebDAV Ref"=w931, "RIO List"=w924, "Valid RIO Connection"=w928, "RIO Folder Found"=w925, "PC Config NOT Saved"=w925) -> (w934:T44)
      }
      frame "WebDAV: Find-RIO-Folder" {
        n275 = Unbundle By Name(w958) -> ("WebDAV Ref"=w963:T42, "RIO Teams Folder"=w961:string)
        n276 = call <vilib>:"Path Info.vi"("session handle"=w963, "relative uri"=w961) -> ("session handle out"=w962:T42, "error out"=w959:errorcluster)  [unwired: 10 in, 2 out]
        n277 = case shown="Error .." w959 {
          tunnel: [w968 w972] -> w964
          tunnel: w962 -> [w968 w975]
          tunnel: w961 -> [_ w971]
          tunnel: [TRUE w969] -> w960
          tunnel: [_ w974] -> _
          frame No Error {
          }
          frame Error {
            n278 = call <vilib>:"Create Directory.vi"("session handle"=w975, "relative uri"=w971) -> ("session handle out"=w973:T42, "error out"=w974:errorcluster)  [unwired: 12 in]
            n279 = call <vilib>:"Path Info.vi"("session handle"=w973, "relative uri"=w971) -> ("session handle out"=w972:T42, "error out"=w970:errorcluster)  [unwired: 10 in, 2 out]
            n280 = Not(x=w970) -> (.not. x?=w969:bool)
          }
        }
        n281 = Bundle By Name(cluster=w958, "WebDAV Ref"=w964, "RIO Folder Found"=w960) -> (w957:T44)
      }
      frame "WebDAV: Get-RIO-FileList" {
        n282 = Unbundle By Name(w982) -> ("WebDAV Ref"=w981:T42, "RIO Teams Folder"=w979:string)
        n283 = call <vilib>:"Directory Listing.vi"("session handle"=w981, "relative uri"=w979, "error in (no error)"=w976) -> ("session handle out"=w980:T42, "file list"=w978:T41[], "error out"=w977:errorcluster)  [unwired: 9 in, 1 out]
        n284 = Bundle By Name(cluster=w982, "WebDAV Ref"=w980, "RIO List"=w978) -> (w983:T44)
      }
      frame "File: Get-PC-FileList" {
        n285 = Unbundle By Name(w987) -> ("PC Path"=w988:path)
        n286 = List Folder(path=w988, pattern="*.cfg") -> (filenames=w986:string[])  [unwired: 2 in, 3 out]
        n287 = Bundle By Name(cluster=w987, "PC file list"=w986) -> (w989:T44)
      }
      frame "File: R-WConfig" {
        n288 = Match Pattern(string=w998, regular expression="-") -> (before substring=w997:string, after substring=w999:string)  [unwired: 1 in, 2 out]
        n289 = call <vilib>:"Trim Whitespace.vi"("string"=w999) -> ("trimmed string"=w1003:string)  [unwired: 1 in]
        n290 = To Upper Case(1:w1003) -> (0:w1002:string)
        n291 = case shown="\"PC\", Default" w997 {
          tunnel: [TRUE FALSE] -> w992
          frame "RIO" {
          }
          frame "PC", Default {
          }
        }
        n292 = case shown="\"READ\", Default" w1002 {
          tunnel: [FALSE ("Read(f) Write(t)") TRUE ("Read(f) Write(t)")] -> w1001
          frame "READ", Default {
          }
          frame "SAVE", "WRITE" {
          }
        }
        n293 = Unbundle By Name(w996) -> ("Current Tab"=w1004:T11)
        n294 = case shown="\"Auto PC Config\"" w1004 {
          tunnel: w996 -> [w1020 w1046 w1072 w1098 w1124 w1150 w1176 w1202 w1228]
          tunnel: [w1021 w1047 w1073 w1099 w1125 w1151 w1177 w1203 w1229] -> w995
          tunnel: w1005 -> [w1018 w1044 w1070 w1096 w1122 w1148 w1174 w1200 w1226]
          tunnel: [w1019 w1045 w1071 w1097 w1123 w1149 w1175 w1201 w1227] -> w993
          tunnel: w1001 -> [w1017 w1043 w1069 w1095 w1121 w1147 w1173 w1199 w1225]
          tunnel: w992 -> [w1016 w1042 w1068 w1094 w1120 w1146 w1172 w1198 w1224]
          frame "Azimuth Config" {
            n295 = case shown="False" w1016 {
              tunnel: [w1032 w1041] -> w1021
              tunnel: w1020 -> [w1031 w1040]
              tunnel: [w1028 w1033] -> w1019
              tunnel: w1018 -> [w1027 w1037]
              tunnel: w1017 -> [w1026 w1036]
              frame True {
                # "RIO"
                n296 = Unbundle By Name(w1031) -> ("WebDAV Ref"=w1025:T42, "RIO Azimuth Config"=w1030:T15, "RIO Teams Folder"=w1022:string)
                n297 = call "RWA_WebDav Config.vim"("Read(f) Write(t)"=w1026, "Session Handle"=w1025, "Error"=w1027, "Reletive Uri Folder"=w1022, "Any Config"=w1030) -> ("Error Out"=w1028:errorcluster, "Message Out"=w1023:string, "Any Config Out"=w1029:T15, "Session Handle Out"=w1024:T42)  [unwired: 2 in, 1 out]
                n298 = Bundle By Name(cluster=w1031, "WebDAV Ref"=w1024, "RIO Azimuth Config"=w1029, "Message"=w1023) -> (w1032:T44)
              }
              frame False {
                # "PC"
                n299 = Unbundle By Name(w1040) -> ("PC Path"=w1035:path, "PC Azimuth Config"=w1039:T15)
                n300 = call "RWA_File Config.vim"("Read(f) Write(t)"=w1036, "Target Folder Folder"=w1035, "Error"=w1037, "Any Config"=w1039) -> ("Error Out"=w1033:errorcluster, "Message Out"=w1034:string, "Any Config Out"=w1038:T15)  [unwired: 3 in, 2 out]
                n301 = Bundle By Name(cluster=w1040, "PC Azimuth Config"=w1038, "Message"=w1034) -> (w1041:T44)
              }
            }
          }
          frame "ExtendProgram Config" {
            n302 = case shown="True" w1042 {
              tunnel: [w1058 w1067] -> w1047
              tunnel: w1046 -> [w1057 w1066]
              tunnel: [w1054 w1063] -> w1045
              tunnel: w1044 -> [w1053 w1062]
              tunnel: w1043 -> [w1052 w1061]
              frame True {
                # "RIO"
                n303 = Unbundle By Name(w1057) -> ("WebDAV Ref"=w1051:T42, "RIO ConeStabber Config"=w1056:T37, "RIO Teams Folder"=w1048:string)
                n304 = call "RWA_WebDav Config.vim"("Read(f) Write(t)"=w1052, "Session Handle"=w1051, "Error"=w1053, "Reletive Uri Folder"=w1048, "Any Config"=w1056) -> ("Error Out"=w1054:errorcluster, "Message Out"=w1049:string, "Any Config Out"=w1055:T37, "Session Handle Out"=w1050:T42)  [unwired: 2 in, 1 out]
                n305 = Bundle By Name(cluster=w1057, "WebDAV Ref"=w1050, "PC ConeStabber Config"=w1055, "Message"=w1049) -> (w1058:T44)
              }
              frame False {
                # "PC"
                n306 = Unbundle By Name(w1066) -> ("PC Path"=w1060:path, "PC ConeStabber Config"=w1065:T37)
                n307 = call "RWA_File Config.vim"("Read(f) Write(t)"=w1061, "Target Folder Folder"=w1060, "Error"=w1062, "Any Config"=w1065) -> ("Error Out"=w1063:errorcluster, "Message Out"=w1059:string, "Any Config Out"=w1064:T37)  [unwired: 3 in, 2 out]
                n308 = Bundle By Name(cluster=w1066, "PC ConeStabber Config"=w1064, "Message"=w1059) -> (w1067:T44)
              }
            }
          }
          frame "Grabber Config" {
            n309 = case shown="True" w1068 {
              tunnel: [w1084 w1093] -> w1073
              tunnel: w1072 -> [w1083 w1092]
              tunnel: [w1080 w1089] -> w1071
              tunnel: w1070 -> [w1079 w1088]
              tunnel: w1069 -> [w1078 w1087]
              frame True {
                # "RIO"
                n310 = Unbundle By Name(w1083) -> ("WebDAV Ref"=w1077:T42, "RIO Grabber Config"=w1082:T38, "RIO Teams Folder"=w1074:string)
                n311 = call "RWA_WebDav Config.vim"("Read(f) Write(t)"=w1078, "Session Handle"=w1077, "Error"=w1079, "Reletive Uri Folder"=w1074, "Any Config"=w1082) -> ("Error Out"=w1080:errorcluster, "Message Out"=w1075:string, "Any Config Out"=w1081:T38, "Session Handle Out"=w1076:T42)  [unwired: 2 in, 1 out]
                n312 = Bundle By Name(cluster=w1083, "WebDAV Ref"=w1076, "RIO Grabber Config"=w1081, "Message"=w1075) -> (w1084:T44)
              }
              frame False {
                # "PC"
                n313 = Unbundle By Name(w1092) -> ("PC Path"=w1086:path, "PC Grabber Config"=w1091:T38)
                n314 = call "RWA_File Config.vim"("Read(f) Write(t)"=w1087, "Target Folder Folder"=w1086, "Error"=w1088, "Any Config"=w1091) -> ("Error Out"=w1089:errorcluster, "Message Out"=w1085:string, "Any Config Out"=w1090:T38)  [unwired: 3 in, 2 out]
                n315 = Bundle By Name(cluster=w1092, "PC Grabber Config"=w1090, "Message"=w1085) -> (w1093:T44)
              }
            }
          }
          frame "Auto PC Config" {
            n316 = case shown="True" w1094 {
              tunnel: [w1110 w1119] -> w1099
              tunnel: w1098 -> [w1109 w1118]
              tunnel: [w1106 w1115] -> w1097
              tunnel: w1096 -> [w1105 w1114]
              tunnel: w1095 -> [w1104 w1113]
              frame True {
                # "RIO"
                n317 = Unbundle By Name(w1109) -> ("WebDAV Ref"=w1103:T42, "RIO Grabber Config"=w1108:T38, "RIO Teams Folder"=w1100:string)
                n318 = call "RWA_WebDav Config.vim"("Read(f) Write(t)"=w1104, "Session Handle"=w1103, "Error"=w1105, "Reletive Uri Folder"=w1100, "Any Config"=w1108) -> ("Error Out"=w1106:errorcluster, "Message Out"=w1101:string, "Any Config Out"=w1107:T38, "Session Handle Out"=w1102:T42)  [unwired: 2 in, 1 out]
                n319 = Bundle By Name(cluster=w1109, "WebDAV Ref"=w1102, "RIO Grabber Config"=w1107, "Message"=w1101) -> (w1110:T44)
              }
              frame False {
                # "PC"
                n320 = Unbundle By Name(w1118) -> ("PC Path"=w1112:path, "PC Grabber Config"=w1117:T38)
                n321 = call "RWA_File Config.vim"("Read(f) Write(t)"=w1113, "Target Folder Folder"=w1112, "Error"=w1114, "Any Config"=w1117) -> ("Error Out"=w1115:errorcluster, "Message Out"=w1111:string, "Any Config Out"=w1116:T38)  [unwired: 3 in, 2 out]
                n322 = Bundle By Name(cluster=w1118, "PC Grabber Config"=w1116, "Message"=w1111) -> (w1119:T44)
              }
            }
          }
          frame "Wrist Config" {
            n323 = case shown="True" w1120 {
              tunnel: [w1136 w1145] -> w1125
              tunnel: w1124 -> [w1135 w1144]
              tunnel: [w1132 w1141] -> w1123
              tunnel: w1122 -> [w1131 w1140]
              tunnel: w1121 -> [w1130 w1139]
              frame True {
                # "RIO"
                n324 = Unbundle By Name(w1135) -> ("WebDAV Ref"=w1129:T42, "RIO Wrist Config"=w1134:T36, "RIO Teams Folder"=w1126:string)
                n325 = call "RWA_WebDav Config.vim"("Read(f) Write(t)"=w1130, "Session Handle"=w1129, "Error"=w1131, "Reletive Uri Folder"=w1126, "Any Config"=w1134) -> ("Error Out"=w1132:errorcluster, "Message Out"=w1127:string, "Any Config Out"=w1133:T36, "Session Handle Out"=w1128:T42)  [unwired: 2 in, 1 out]
                n326 = Bundle By Name(cluster=w1135, "WebDAV Ref"=w1128, "RIO Wrist Config"=w1133, "Message"=w1127) -> (w1136:T44)
              }
              frame False {
                # "PC"
                n327 = Unbundle By Name(w1144) -> ("PC Path"=w1138:path, "PC Wrist Config"=w1143:T36)
                n328 = call "RWA_File Config.vim"("Read(f) Write(t)"=w1139, "Target Folder Folder"=w1138, "Error"=w1140, "Any Config"=w1143) -> ("Error Out"=w1141:errorcluster, "Message Out"=w1137:string, "Any Config Out"=w1142:T36)  [unwired: 3 in, 2 out]
                n329 = Bundle By Name(cluster=w1144, "PC Wrist Config"=w1142, "Message"=w1137) -> (w1145:T44)
              }
            }
          }
          frame "ExtendFX Config" {
            n330 = case shown="True" w1146 {
              tunnel: [w1162 w1171] -> w1151
              tunnel: w1150 -> [w1161 w1170]
              tunnel: [w1158 w1167] -> w1149
              tunnel: w1148 -> [w1157 w1166]
              tunnel: w1147 -> [w1156 w1165]
              frame True {
                # "RIO"
                n331 = Unbundle By Name(w1161) -> ("WebDAV Ref"=w1155:T42, "RIO Extender Config"=w1160:T34, "RIO Teams Folder"=w1152:string)
                n332 = call "RWA_WebDav Config.vim"("Read(f) Write(t)"=w1156, "Session Handle"=w1155, "Error"=w1157, "Reletive Uri Folder"=w1152, "Any Config"=w1160) -> ("Error Out"=w1158:errorcluster, "Message Out"=w1153:string, "Any Config Out"=w1159:T34, "Session Handle Out"=w1154:T42)  [unwired: 2 in, 1 out]
                n333 = Bundle By Name(cluster=w1161, "WebDAV Ref"=w1154, "RIO Extender Config"=w1159, "Message"=w1153) -> (w1162:T44)
              }
              frame False {
                # "PC"
                n334 = Unbundle By Name(w1170) -> ("PC Path"=w1164:path, "PC Extender Config"=w1169:T34)
                n335 = call "RWA_File Config.vim"("Read(f) Write(t)"=w1165, "Target Folder Folder"=w1164, "Error"=w1166, "Any Config"=w1169) -> ("Error Out"=w1167:errorcluster, "Message Out"=w1163:string, "Any Config Out"=w1168:T34)  [unwired: 3 in, 2 out]
                n336 = Bundle By Name(cluster=w1170, "PC Extender Config"=w1168, "Message"=w1163) -> (w1171:T44)
              }
            }
          }
          frame "Sholder Config" {
            n337 = case shown="True" w1172 {
              tunnel: [w1188 w1197] -> w1177
              tunnel: w1176 -> [w1187 w1196]
              tunnel: [w1184 w1193] -> w1175
              tunnel: w1174 -> [w1183 w1192]
              tunnel: w1173 -> [w1182 w1191]
              frame True {
                # "RIO"
                n338 = Unbundle By Name(w1187) -> ("WebDAV Ref"=w1181:T42, "RIO Sholder Config"=w1186:T26, "RIO Teams Folder"=w1178:string)
                n339 = call "RWA_WebDav Config.vim"("Read(f) Write(t)"=w1182, "Session Handle"=w1181, "Error"=w1183, "Reletive Uri Folder"=w1178, "Any Config"=w1186) -> ("Error Out"=w1184:errorcluster, "Message Out"=w1179:string, "Any Config Out"=w1185:T26, "Session Handle Out"=w1180:T42)  [unwired: 2 in, 1 out]
                n340 = Bundle By Name(cluster=w1187, "WebDAV Ref"=w1180, "RIO Sholder Config"=w1185, "Message"=w1179) -> (w1188:T44)
              }
              frame False {
                # "PC"
                n341 = Unbundle By Name(w1196) -> ("PC Path"=w1190:path, "PC Sholder Config"=w1195:T26)
                n342 = call "RWA_File Config.vim"("Read(f) Write(t)"=w1191, "Target Folder Folder"=w1190, "Error"=w1192, "Any Config"=w1195) -> ("Error Out"=w1193:errorcluster, "Message Out"=w1189:string, "Any Config Out"=w1194:T26)  [unwired: 3 in, 2 out]
                n343 = Bundle By Name(cluster=w1196, "PC Sholder Config"=w1194, "Message"=w1189) -> (w1197:T44)
              }
            }
          }
          frame "Drive Config" {
            n344 = case shown="True" w1198 {
              tunnel: [w1214 w1223] -> w1203
              tunnel: w1202 -> [w1213 w1222]
              tunnel: [w1210 w1219] -> w1201
              tunnel: w1200 -> [w1209 w1218]
              tunnel: w1199 -> [w1208 w1217]
              frame True {
                # "RIO"
                n345 = Unbundle By Name(w1213) -> ("WebDAV Ref"=w1207:T42, "RIO Drive Config"=w1212:T24, "RIO Teams Folder"=w1204:string)
                n346 = call "RWA_WebDav Config.vim"("Read(f) Write(t)"=w1208, "Session Handle"=w1207, "Error"=w1209, "Reletive Uri Folder"=w1204, "Any Config"=w1212) -> ("Error Out"=w1210:errorcluster, "Message Out"=w1205:string, "Any Config Out"=w1211:T24, "Session Handle Out"=w1206:T42)  [unwired: 2 in, 1 out]
                n347 = Bundle By Name(cluster=w1213, "WebDAV Ref"=w1206, "RIO Drive Config"=w1211, "Message"=w1205) -> (w1214:T44)
              }
              frame False {
                # "PC"
                n348 = Unbundle By Name(w1222) -> ("PC Path"=w1216:path, "PC Drive Config"=w1221:T24)
                n349 = call "RWA_File Config.vim"("Read(f) Write(t)"=w1217, "Target Folder Folder"=w1216, "Error"=w1218, "Any Config"=w1221) -> ("Error Out"=w1219:errorcluster, "Message Out"=w1215:string, "Any Config Out"=w1220:T24)  [unwired: 3 in, 2 out]
                n350 = Bundle By Name(cluster=w1222, "PC Drive Config"=w1220, "Message"=w1215) -> (w1223:T44)
              }
            }
          }
          frame "Module Specific" {
            n351 = case shown="False" w1224 {
              tunnel: [w1240 w1249] -> w1229
              tunnel: w1228 -> [w1239 w1248]
              tunnel: [w1236 w1245] -> w1227
              tunnel: w1226 -> [w1235 w1244]
              tunnel: w1225 -> [w1234 w1243]
              frame True {
                # "RIO"
                n352 = Unbundle By Name(w1239) -> ("WebDAV Ref"=w1233:T42, "RIO Module Specific Data"=w1238:T12, "RIO Teams Folder"=w1230:string)
                n353 = call "RWA_WebDav Config.vim"("Read(f) Write(t)"=w1234, "Session Handle"=w1233, "Error"=w1235, "Reletive Uri Folder"=w1230, "Any Config"=w1238) -> ("Error Out"=w1236:errorcluster, "Message Out"=w1231:string, "Any Config Out"=w1237:T12, "Session Handle Out"=w1232:T42)  [unwired: 2 in, 1 out]
                n354 = Bundle By Name(cluster=w1239, "WebDAV Ref"=w1232, "RIO Module Specific Data"=w1237, "Message"=w1231) -> (w1240:T44)
              }
              frame False {
                # "PC"
                n355 = Unbundle By Name(w1248) -> ("PC Path"=w1242:path, "PC Module Specific Data"=w1247:T12)
                n356 = call "RWA_File Config.vim"("Read(f) Write(t)"=w1243, "Target Folder Folder"=w1242, "Error"=w1244, "Any Config"=w1247) -> ("Error Out"=w1245:errorcluster, "Message Out"=w1241:string, "Any Config Out"=w1246:T12)  [unwired: 3 in, 2 out]
                n357 = Bundle By Name(cluster=w1248, "PC Module Specific Data"=w1246, "Message"=w1241) -> (w1249:T44)
              }
            }
          }
        }
        n358 = case shown="False" w992 {
          tunnel: w995 -> [w1010 w1011]
          tunnel: [w1009 w1011] -> w994
          tunnel: w993 -> [w1008 _]
          frame False {
            n359 = Unbundle By Name(w1008) -> ("status"=w1007:bool)
            n360 = Bundle By Name(cluster=w1010, "PC Config NOT Saved"=w1007) -> (w1009:T44)
          }
          frame True {
          }
        }
      }
    }
    n361 = Unbundle By Name(w57) -> ("RIO IP List"=w70:string[], "IP Index"=w68:i32)
    n362 = Unbundle By Name(w57) -> ("Current Tab"=w55:T11)
    n363 = Unbundle By Name(w57) -> ("Message"=→"Message":string, "Valid RIO Connection"=→"RIO Connected":bool, "RIO Folder Found"=→"RIO Folder Found":bool, "PC Folder Found"=→"PC Folder Found":bool)
    n364 = call "Is Value Changed.vim"("value"=w70) -> ("changed or first call?"=w66:bool)
    n365 = call "Is Value Changed.vim"("value"=w68) -> ("changed or first call?"=w69:bool)
    n366 = Unbundle By Name(w57) -> ("State"=→"State":T40, "RIO url"=w62:string, "PC Path"=→"PC Folder Path":path)
    n367 = case shown="\"Grabber Config\"" w55 {
      tunnel: w57 -> [w307 w313 w319 w325 w331 w337 w343 w349]
      tunnel: [w303 w310 w317 w323 w329 w335 w341 w347] -> w58
      frame "Azimuth Config" {
        n368 = Unbundle By Name(w307) -> ("PC Azimuth Config"=w304:T15, "RIO Azimuth Config"=w305:T15)
        "RIO Azimuth Config Data" <- w305
        n369 = call "Is Value Changed.vim"("value"=w304) -> ("changed or first call?"=w306:bool)
        n370 = Not Equal?(x=w304, y=w305) -> (x != y?=w303:bool)
        n371 = case shown="False" w306 {
          tunnel: w304 -> [_ w308]
          frame False {
          }
          frame True {
            n372 = local write "PC Azimuth Config Data"(w308) -> ()
          }
        }
      }
      frame "Drive Config" {
        n373 = Unbundle By Name(w313) -> ("PC Drive Config"=w311:T24, "RIO Drive Config"=w309:T24)
        "RIO Drive Config Data" <- w309
        n374 = call "Is Value Changed.vim"("value"=w311) -> ("changed or first call?"=w312:bool)
        n375 = Not Equal?(x=w311, y=w309) -> (x != y?=w310:bool)
        n376 = case shown="True" w312 {
          tunnel: w311 -> [_ w314]
          frame False {
          }
          frame True {
            n377 = local write "PC Drive Config Data"(w314) -> ()
          }
        }
      }
      frame "Sholder Config" {
        n378 = Unbundle By Name(w319) -> ("PC Sholder Config"=w315:T26, "RIO Sholder Config"=w316:T26)
        "RIO Sholder Config" <- w316
        n379 = call "Is Value Changed.vim"("value"=w315) -> ("changed or first call?"=w318:bool)
        n380 = Not Equal?(x=w315, y=w316) -> (x != y?=w317:bool)
        n381 = case shown="True" w318 {
          tunnel: w315 -> [_ w320]
          frame False {
          }
          frame True {
            n382 = local write "PC Sholder Config"(w320) -> ()
          }
        }
      }
      frame "ExtendFX Config" {
        n383 = Unbundle By Name(w325) -> ("PC Extender Config"=w321:T34, "RIO Extender Config"=w322:T34)
        "RIO Extender Config" <- w322
        n384 = call "Is Value Changed.vim"("value"=w321) -> ("changed or first call?"=w324:bool)
        n385 = Not Equal?(x=w321, y=w322) -> (x != y?=w323:bool)
        n386 = case shown="True" w324 {
          tunnel: w321 -> [_ w326]
          frame False {
          }
          frame True {
            n387 = local write "PC Extend ConfigFX"(w326) -> ()
          }
        }
      }
      frame "Wrist Config" {
        n388 = Unbundle By Name(w331) -> ("PC Wrist Config"=w327:T36, "RIO Wrist Config"=w328:T36)
        "RIO Wrist Config" <- w328
        n389 = call "Is Value Changed.vim"("value"=w327) -> ("changed or first call?"=w330:bool)
        n390 = Not Equal?(x=w327, y=w328) -> (x != y?=w329:bool)
        n391 = case shown="True" w330 {
          tunnel: w327 -> [_ w332]
          frame False {
          }
          frame True {
            n392 = local write "PC Wrist Config"(w332) -> ()
          }
        }
      }
      frame "ExtendProgram Config" {
        n393 = Unbundle By Name(w337) -> ("PC ConeStabber Config"=w333:T37, "RIO ConeStabber Config"=w334:T37)
        "RIO ExtendProgram Config" <- w334
        n394 = call "Is Value Changed.vim"("value"=w333) -> ("changed or first call?"=w336:bool)
        n395 = Not Equal?(x=w333, y=w334) -> (x != y?=w335:bool)
        n396 = case shown="True" w336 {
          tunnel: w333 -> [_ w338]
          frame False {
          }
          frame True {
            n397 = local write "PC ExtendProgram Config"(w338) -> ()
          }
        }
      }
      frame "Grabber Config" {
        n398 = Unbundle By Name(w343) -> ("PC Grabber Config"=w339:T38, "RIO Grabber Config"=w340:T38)
        "RIO Grabber Config" <- w340
        n399 = call "Is Value Changed.vim"("value"=w339) -> ("changed or first call?"=w342:bool)
        n400 = Not Equal?(x=w339, y=w340) -> (x != y?=w341:bool)
        n401 = case shown="True" w342 {
          tunnel: w339 -> [_ w344]
          frame False {
          }
          frame True {
            n402 = local write "PC Grabber Config"(w344) -> ()
          }
        }
      }
      frame "Module Specific" {
        n403 = Unbundle By Name(w349) -> ("PC Module Specific Data"=w345:T12, "RIO Module Specific Data"=w346:T12)
        "RIO Module Specific Data" <- w346
        n404 = call "Is Value Changed.vim"("value"=w345) -> ("changed or first call?"=w348:bool)
        n405 = Not Equal?(x=w345, y=w346) -> (x != y?=w347:bool)
        n406 = case shown="False" w348 {
          tunnel: w345 -> [_ w350]
          frame False {
          }
          frame True {
            n407 = local write "PC Module Specific Data"(w350) -> ()
          }
        }
      }
    }
    "Config NOT Equal" <- w58
    n408 = Or(x=w66, y=w69) -> (x .or. y?=w67:bool)
    n409 = call "Is Value Changed.vim"("value"=w55) -> ("changed or first call?"=w59:bool)
    n410 = case shown="False" w66 {
      tunnel: w70 -> [_ w360]
      frame False {
      }
      frame True {
        n411 = local write "RIO IP List"(w360) -> ()
      }
    }
    n412 = call "Is Value Changed.vim"("value"=w62) -> ("changed or first call?"=w63:bool)
    n413 = case shown="False" w67 {
      tunnel: w70 -> [_ w359]
      tunnel: w68 -> [_ w355]
      frame False {
      }
      frame True {
        n414 = Array Size(array=w359) -> (size(s)=w358:i32)
        n415 = Initialize Array(FALSE, w358) -> (w356:bool[])
        n416 = Replace Array Subset(array=w356, new element=TRUE ("new element/subarray"), index=w355) -> (w353:bool[])
        n417 = local write "Select"(w353) -> ()
      }
    }
    n418 = case shown="False" w59 {
      tunnel: w55 -> [_ w351]
      frame False {
      }
      frame True {
        n419 = local write "Config Tab"(w351) -> ()
      }
    }
    n420 = case shown="False" w63 {
      tunnel: w62 -> [_ w352]
      frame False {
      }
      frame True {
        n421 = local write "RIO Folder Path"(w352) -> ()
      }
    }
    n422 = Unbundle By Name(w57) -> ("PC Config NOT Saved"=→"PC Config NOT Saved":bool)
  }
  n423 = disable-structure shown="Disabled" {
    frame Disabled {
      (unwired) ENUM_Request_PC_File_Manager."None <<Process State>>"  # Request
      (unwired) ENUM_State_PC_File_Manager."<Startup>"  # State
    }
    frame Enabled {
    }
  }
  n424 = disable-structure shown="Enabled" {
    frame Disabled {
      (unwired) ENUM_Request_PC_File_Manager."Stop Program"  # Requests
      (unwired) ENUM_State_PC_File_Manager."Waiting for Connection"  # State
      n425 = call "Add State(s) to state machine.vi"() -> ()  [unwired: 15 in, 1 out]
    }
    frame Enabled {
    }
  }
  n426 = flat-sequence {
    tunnel: w7 -> [w1253]
    tunnel: w6 -> [_]
    tunnel: w5 -> [_]
    frame #0 {
      n427 = Unbundle By Name(w1253) -> ("This VI"=w1251:refnum<vi>, "FP Data"=w1252:refnum<class "DecFrame_FP.lvclass">)
      n428 = call-dynamic "Set State.vi"("VI Ref"=w1251, "State"=T46."Closed", "FP"=w1252) -> ()  [unwired: 6 in, 3 out]
    }
  }
